vi "Microscope_control-illumination_camera_Galvo_EOM.vi"() -> ()   [LabVIEW 2012]
uses:
  <vilib>/Utility/error.llb/DialogType.ctl
  <vilib>/DAQmx/read.llb/DAQmx Read (Analog DBL 1Chan 1Samp).vi
  <vilib>/DAQmx/write.llb/DAQmx Write (Digital 1D Bool NChan 1Samp 1Line).vi
  <vilib>/DAQmx/write.llb/DAQmx Write (Analog 1D DBL NChan 1Samp).vi
  <vilib>/DAQmx/read.llb/DAQmx Read (Analog 2D DBL NChan NSamp).vi
  <vilib>/DAQmx/write.llb/DAQmx Write (Analog 1D Wfm NChan NSamp).vi
  <vilib>/DAQmx/write.llb/DAQmx Write (Analog DBL 1Chan 1Samp).vi
  <vilib>/DAQmx/create/channels.llb/DAQmx Create Channel (AI-Voltage-Basic).vi
  <vilib>/DAQmx/miscellaneous.llb/DAQmx Fill In Error Info.vi
  <vilib>/addons/control/pid/pid.llb/PID Advanced (DBL).vi
  <vilib>/DAQmx/create/channels.llb/DAQmx Create Channel (DO-Digital Output).vi
  <vilib>/DAQmx/create/channels.llb/DAQmx Create Channel (AO-Voltage-Basic).vi
  <vilib>/Analysis/baseanly.llb/Mean (DBL).vi
  <vilib>/DAQmx/configure/timing.llb/DAQmx Timing (Use Waveform).vi
  <vilib>/Analysis/NI_AALBase.lvlib
  <instrlib>/Olympus IX BX Series/Olympus IX BX Series.lvlib
  <vilib>/addons/control/pid/NI_PID_pid.lvlib
panel:
  in  "Laser Trig 1":bool
  in  "# repeats":i16=6
  in  "Splice?":bool
  in  "Digital  Time Step":dbl=0.0005 format="%.4f"
  in  "Synced Trigger?":bool
  out "Digital Waveform":digitalwaveform[](graph)=[{"t0"=timestamp(0 s since 1904-01-01), "dt"=0.0, "Y"={"transitions"=[0, 2, 30, 32, 60, 62, 90, 92, 120, 122, 150, 152, 180, 182, 210, 212, 240, 242, 270, 272, 300, 302, 330, 332, 360, 362, 390, 392, 420, 422, 450, 452, 480, 482, 510, 512, 540, 542, 570, 572, 600, 601], "data"=[[1], [0], [1], [0], [1], [0], [1], [0], [1], [0], [1], [0], [1], [0], [1], [0], [1], [0], [1], [0], [1], [0], [1], [0], [1], [0], [1], [0], [1], [0], [1], [0], [1], [0], [1], [0], [1], [0], [1], [0], [1], [0]]}, "error"={"status"=FALSE, "code"=37421928, "source"=""}}, {"t0"=timestamp(0 s since 1904-01-01), "dt"=0.0, "Y"={"transitions"=[0, 11, 21, 41, 51, 71, 81, 101, 111, 131, 141, 161, 171, 191, 201, 221, 231, 251, 261, 281, 291, 311, 321, 341, 351, 371, 381, 401, 411, 431, 441, 461, 471, 491, 501, 521, 531, 551, 561, 581, 591, 601], "data"=[[0], [1], [0], [1], [0], [1], [0], [1], [0], [1], [0], [1], [0], [1], [0], [1], [0], [1], [0], [1], [0], [1], [0], [1], [0], [1], [0], [1], [0], [1], [0], [1], [0], [1], [0], [1], [0], [1], [0], [1], [0], [0]]}, "error"={"status"=FALSE, "code"=37421928, "source"=""}}]
  out "number of samples":i32=602
  in  "CO.Pulse.Term":tag="/Dev2/PFI0"
  in  "Cycle time":dbl=30.0 format="%.4f"
  out "Clock Rate":dbl=66666.66666666667
  in  "Digital lines":tag="Dev2/port0/line8:9"
  in  "Digital Data":digitalwaveform[](array[waveform])=[{"t0"=timestamp(0 s since 1904-01-01), "dt"=0.0, "Y"={"transitions"=[0, 2, 30, 32, 60, 62, 90, 92, 120, 122, 150, 152, 180, 182, 210, 212, 240, 242, 270, 272, 300, 302, 330, 332, 360, 362, 390, 392, 420, 422, 450, 452, 480, 482, 510, 512, 540, 542, 570, 572, 600, 601], "data"=[[1], [0], [1], [0], [1], [0], [1], [0], [1], [0], [1], [0], [1], [0], [1], [0], [1], [0], [1], [0], [1], [0], [1], [0], [1], [0], [1], [0], [1], [0], [1], [0], [1], [0], [1], [0], [1], [0], [1], [0], [1], [0]]}, "error"={"status"=FALSE, "code"=37421928, "source"=""}}, {"t0"=timestamp(0 s since 1904-01-01), "dt"=0.0, "Y"={"transitions"=[0, 11, 21, 41, 51, 71, 81, 101, 111, 131, 141, 161, 171, 191, 201, 221, 231, 251, 261, 281, 291, 311, 321, 341, 351, 371, 381, 401, 411, 431, 441, 461, 471, 491, 501, 521, 531, 551, 561, 581, 591, 601], "data"=[[0], [1], [0], [1], [0], [1], [0], [1], [0], [1], [0], [1], [0], [1], [0], [1], [0], [1], [0], [1], [0], [1], [0], [1], [0], [1], [0], [1], [0], [1], [0], [1], [0], [1], [0], [1], [0], [1], [0], [1], [0], [0]]}, "error"={"status"=FALSE, "code"=37421928, "source"=""}}]
  in  "counter ch. #":tag="Dev2/ctr0"
  out "Array":dbl[](array[numeric])=[5.218535567851096e-05]
  in  "Quiver full amp":dbl=10.0 min=0.0 max=360.0 format="%0.1p"
  in  "W-E Phase":dbl format="%.2f"
  in  "Quiver Direction":i32(ring) items=["North", "East", "South", "West"]
  in  "quiver offset":dbl format="%0.2p"
  in  "quiver offset":dbl format="%0.2p"
  in  "EOM spin? (Quiver)":bool
  in  "Phase":dbl format="%.2f"
  in  "Phase":dbl step=0.1 format="%.2f"
  in  "Offset":dbl min=-1.0 max=1.0 step=0.001 format="%.3f"
  in  "Offset":dbl min=-1.0 max=1.0 format="%.3f"
  out "Quivering":bool
  in  "180° Shift":bool
  in  "180° Shift":bool
  in  "Quiver":bool
  in  "180° Shift":bool
  in  "180° Shift (s)":bool
  in  "Center exclude":dbl=0.1
  in  "E/W EOM":dbl=0.07
  in  "N/S EOM":dbl=0.07
  in  "EOM spin?":bool=TRUE
  in  "EOM Voltage (Ch. 3)":dbl(slide) step=0.0001 scale=-0.7..0.7 scale format="%#_4g"
  out "Direction":u16(ring) items=["", "North", "East", "South", "West", "Spin", "Sync"]
  in  "Center":bool
  in  "South":bool
  in  "East":bool
  in  "West":bool
  in  "North":bool
  in  "output range":cluster{"out high":dbl, "out low":dbl}={"out high"=1.0, "out low"=-1.0} {"out low" format="%.2f"; "out high" format="%.2f"}
  in  "Lock-in Amp In":tag="Dev2/ai16" caption="Lock In Detect In"
  in  "Focus Position?":bool
  out "position (um)":T1(graph)={"data"=-0.13365967335514356, "position (um)"=7583.27, "element"=0.0}
  in  "Use current position?":bool
  in  "setpoint range":cluster{"SP high":dbl, "SP low":dbl}={"SP high"=5.0, "SP low"=-5.0} {"SP high" format="%.2f"; "SP low" format="%.2f"}
  out "Notification":u16(ring) items=["", "Spin must be activated for focus lock", "Spin must be activated for focus detection", "Disable EOM spin"]
  in  "Lock Z":bool
  in  "Focus limit width":dbl=1000.0
  in  "Focus Limit Center":dbl=7500.0 format="%.1f"
  in  "IX2-UCB port":refnum<visa-resource-name>="COM1"
  in  "Sampling Time":dbl=100.0 format="%.2f"
  in  "PID gains":T2={"proportional gain (Kc)"=0.8, "integral time (Ti, min)"=0.0, "derivative time (Td, min)"=0.0} {"derivative time (Td, min)" format="%#.6g"; "integral time (Ti, min)" format="%#.6g"; "proportional gain (Kc)" format="%#.6g"}
  in  "Z lock setpoint (Volt)":dbl(slide) min=-5.0 max=5.0 step=0.01 scale=-5.0..5.0 scale format="%#_4g"
  in  "Write Y/X ration \nduring center find?":bool=TRUE
  out "W-E Width":dbl=0.63 format="%#_5g"
  out "N-S Width":dbl=0.63 format="%#_5g"
  out "Spinning":bool
  in  "Stop spin":bool caption="stop"
  out "output cluster":cluster{dbl, "# sample":i32}={66666.66666666667, "# sample"=2000}
  in  "# sample":i32=2000
  in  "Y/X ration \nW-E = C*(N-S)":dbl=1.0 format="%.3f"
  in  "Amplitude":dbl min=0.0 max=1.0 step=0.001 format="%.3f"
  in  "Amplitude":dbl=-0.54 step=0.001 format="%.3f"
  in  "Offset":dbl min=-1.0 max=1.0 format="%.3f"
  in  "Offset":dbl=-0.135 min=-1.0 max=1.0 step=0.001 format="%.3f"
  out "Output Waveform":waveform(dbl)[](graph)=[{"t0"=timestamp(0 s since 1904-01-01), "dt"=1.4999999999999999e-05, "Y"=array[2000 elements]}, {"t0"=timestamp(0 s since 1904-01-01), "dt"=1.4999999999999999e-05, "Y"=array[2000 elements]}, {"t0"=timestamp(0 s since 1904-01-01), "dt"=1.4999999999999999e-05, "Y"=array[2000 elements]}, {"t0"=timestamp(0 s since 1904-01-01), "dt"=1.4999999999999999e-05, "Y"=array[2000 elements]}]
  in  "Spin Amp (N-S)":dbl=0.68 format="%.3f"
  in  "Phase":dbl step=0.1 format="%.2f"
  in  "Phase":dbl=-70.0 format="%.2f"
  in  "W-E Phase Delay":dbl=90.0 format="%.2g"
  in  "Frequency":dbl=200.0 min=0.0 max=300.0 format="%0.2p"
  in  "Spin":bool
  out "Text Ring":u16(ring)=1 items=["East-West", "North-South"]
  in  "Centering Iterations":i32=4
  in  "2D Center Find":bool
  in  "Y":dbl(slide) scale=1.0..-1.0 scale format="%#.4g"
  in  "X":dbl(slide) scale=-1.0..1.0 scale format="%#.3g"
  out "Manual Control":dbl(knob)=-0.003845687659202201 scale=-0.01..0.2
  in  "Differential Initial Conditions":dbl[](array[numeric])=[-0.005, -0.005] format="%#_6f"
  in  "Scan Galvo Selection":bool
  out "Amplitude":dbl=0.63 format="%#_4g"
  out "Offset":dbl=0.03399999999999992 format="%#_3g"
  out "Right":dbl=0.6639999999999999 format="%#_4g"
  out "left":dbl=-0.5960000000000001 format="%#_4g"
  in  "Differential Method":u16(ring)=1 items=["2nd Order Central", "4th Order Central", "Forward", "Backward"]
  out "X Y Sensor Graph":cluster{"Array":dbl[], "Array":dbl[]}[](graph)
  in  "samples per step":i32=10
  out "Sum Graph":cluster{"Array":dbl[], "dX/dt":dbl[]}[](graph)
  in  "Analog Input Channels":tag="Dev2/ai0:2" caption="Quad Detector In"
  in  "ms to wait":u32
  in  "Steps":i16=1601 caption="scan steps"
  in  "End voltage (scanned galvo)":dbl=0.8 caption="End Scan" format="%0.2f"
  in  "Start voltage (scanned galvo)":dbl=-0.8 caption="Start Scan" format="%0.2f"
  in  "Galvo Hard Max Voltage":dbl=1.0 caption="Max Value" format="%0.2f"
  in  "Galvo Hard Min Voltage":dbl=-1.0 caption="Min Value" format="%0.2f"
  in  "Analog Out Channels":tag="Dev2/ao0:3" caption="Galvo/EOM Out"
  in  "Scan Galvo":bool
  in  "stop":bool
  # "N-S"
  # "E-W"
  # "Channel 3"
  # "Channel 4"
  # "Channel 3"
  # "Channel 4"
  # "Hz"
  # "deg"
  # "V"
  # "deg"
  # "N"
  # "s"
  # "s"
  # "N/S (p), \nE/W (s)"
  # "N/S (s), \nE/W (p)"
  # "W"
  # "E"
  # "S"
  # "V"
  # "V"
  # "N/S (p), \nE/W (s)"
  # "DAQ Parameters"
  # "ms"
  # "nm"
  # "nm"
  # "Center Scan Parameters"
  # "V"
  # "V"
  # "V"
  # "ms"
  # "V"
  # "Notes: Analog Output Ch. 1 and 2 designed to control two axis of galvonometers, Ch.3 and 4 are for EOM. \nCh.1 and 2 consists of sine wave, typically with relative phase shift of ~90 deg, to generate a circular scan\nCh. 3 and 4 are sawtooth scans at twice frequency of Ch. 1 and 2.  \n2D centerfind detects X and Y axis TIR conditions (from back reflection detector), in order to find beam center position for circle scanning\nParameters on upper right panels are for sending TTL pulses/triggers to lasers/cameras/flow valves.  Ch. 1-4 analog outputs (for galvos and EOM) can be synced with this TTL triggers\nParameters on lower right are for controlling microscope focus feedback using back reflection detector (Olympus IX2 series)."
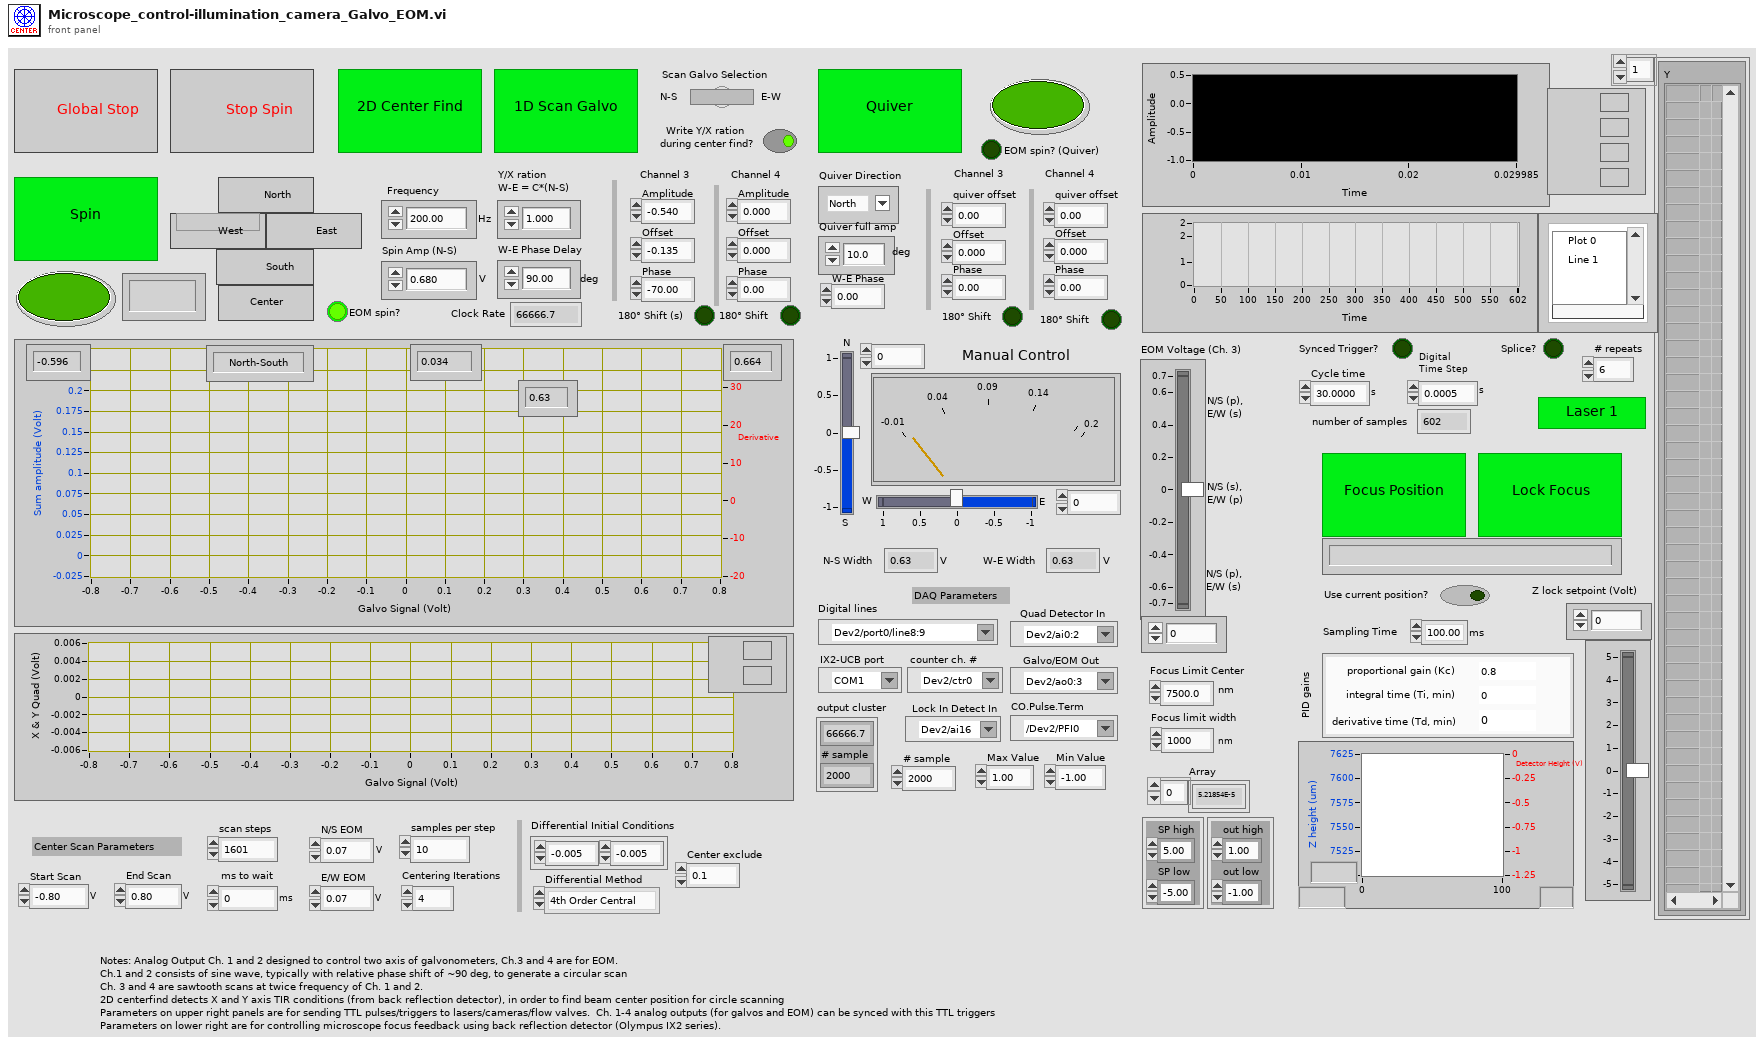
[diagram p1: front panel]
types:
  T1 = cluster{"data":dbl, "position (um)":dbl, "element":dbl}
  T2 = cluster{"proportional gain (Kc)":dbl, "integral time (Ti, min)":dbl, "derivative time (Td, min)":dbl}
  T3 = typedef "DialogType.ctl" = u16
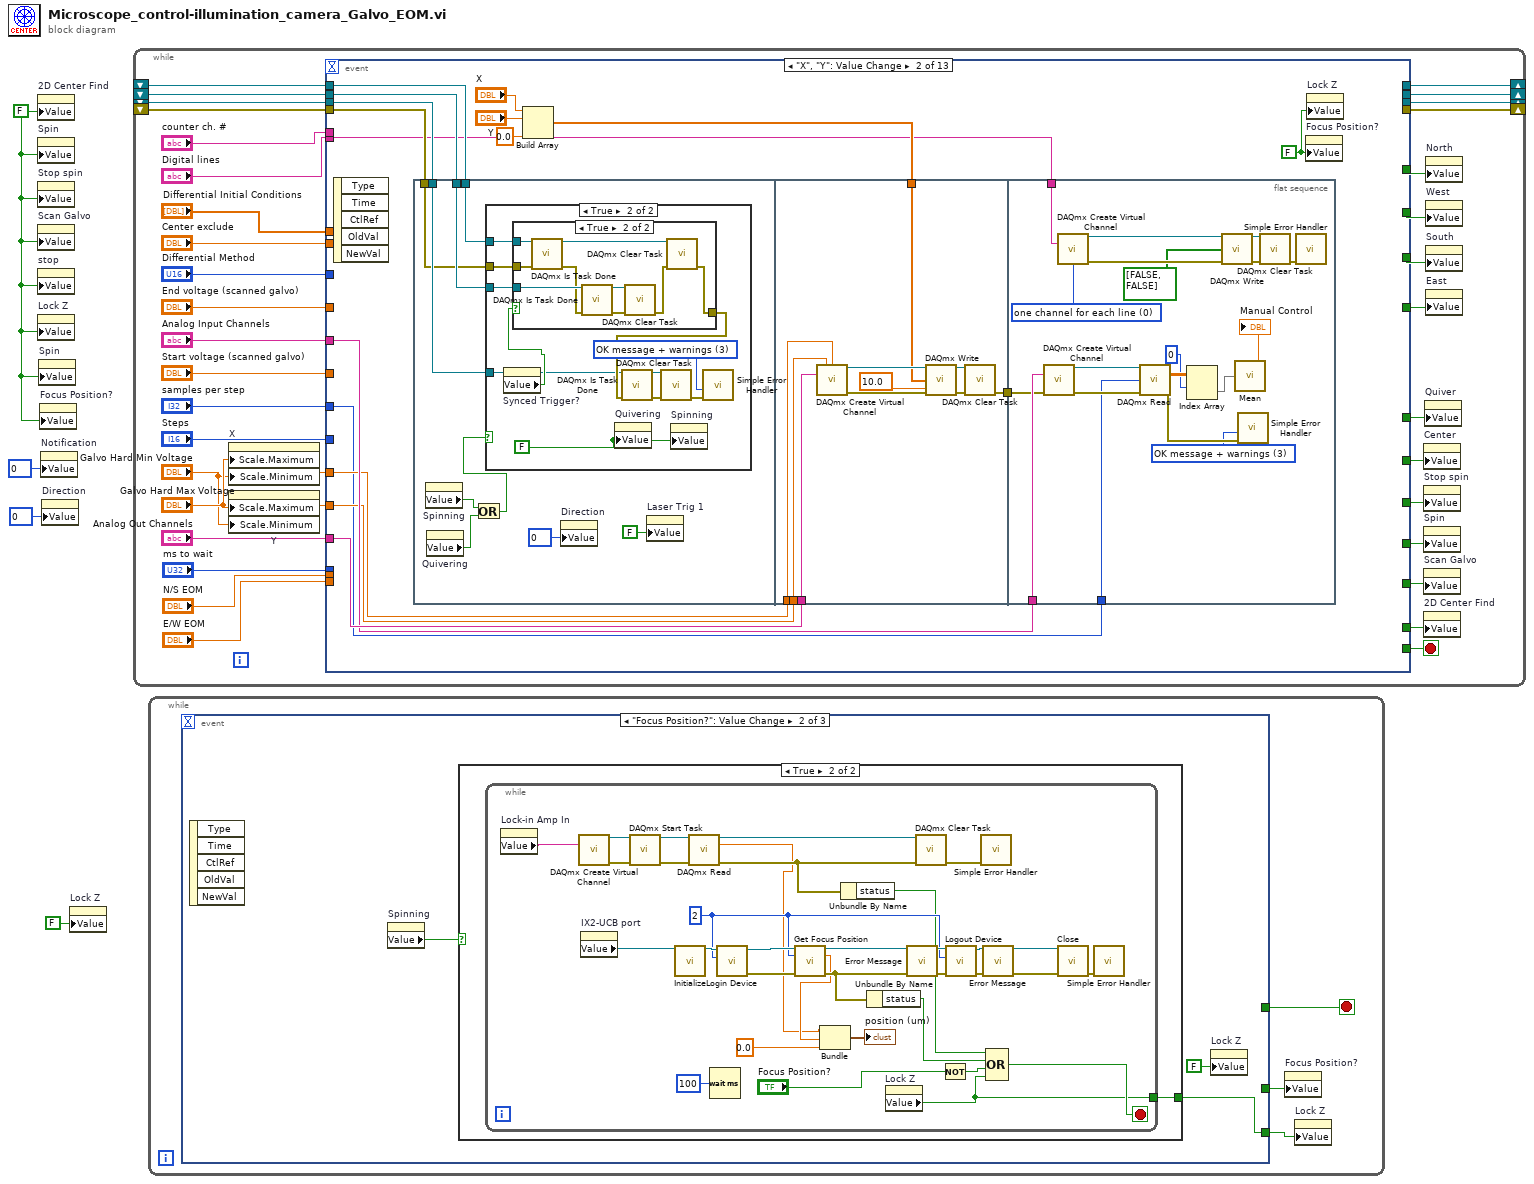
[diagram p0: block diagram]
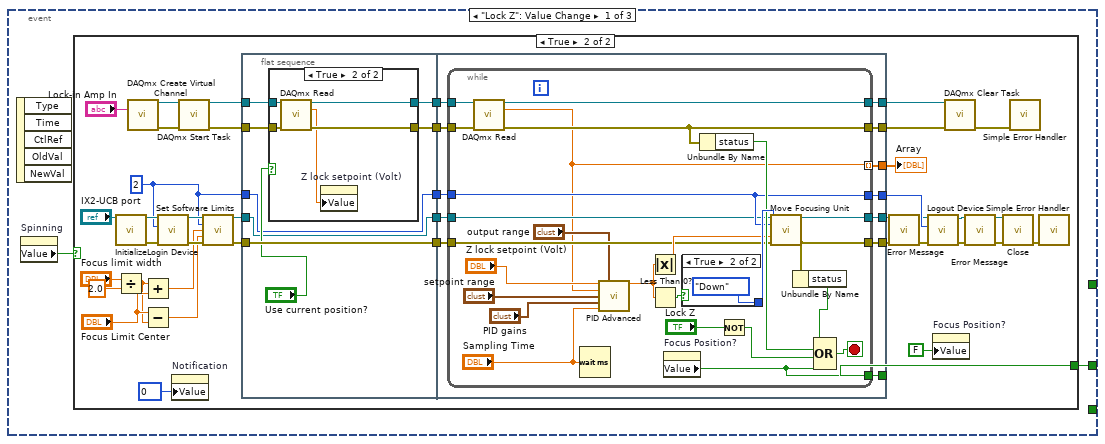
[diagram p2: hidden frame]
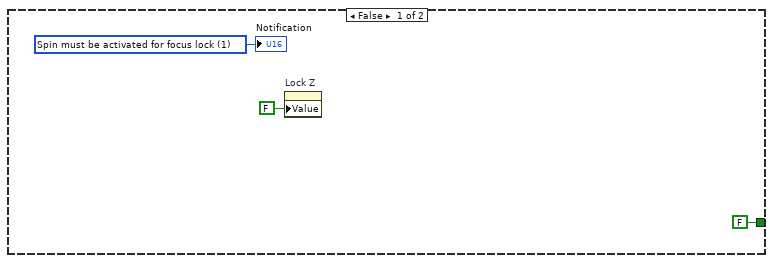
[diagram p3: hidden frame]
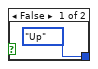
[diagram p5: hidden frame]
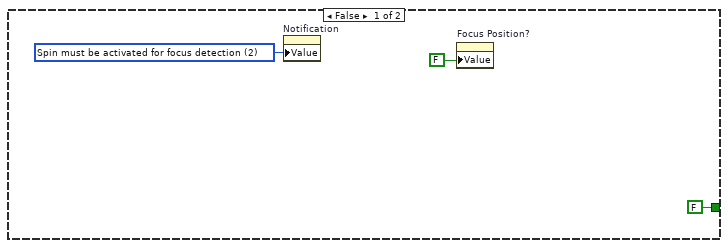
[diagram p6: hidden frame]
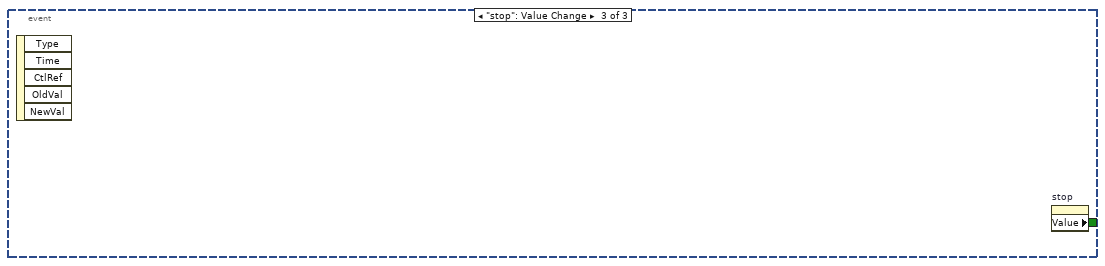
[diagram p7: hidden frame]
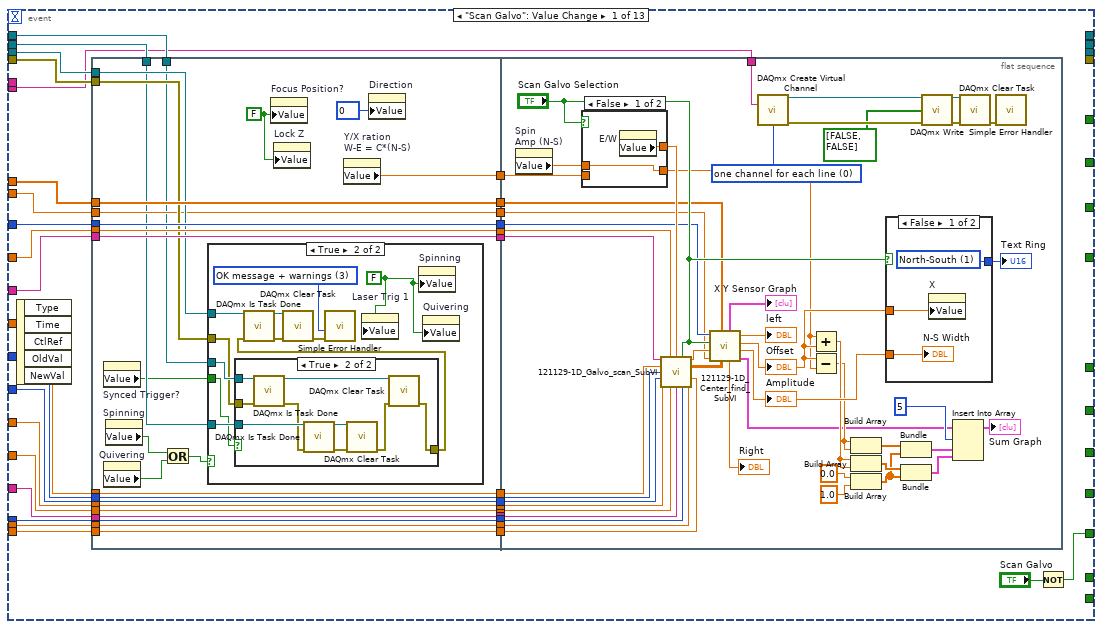
[diagram p8: hidden frame]
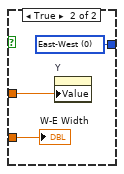
[diagram p11: hidden frame]
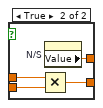
[diagram p12: hidden frame]
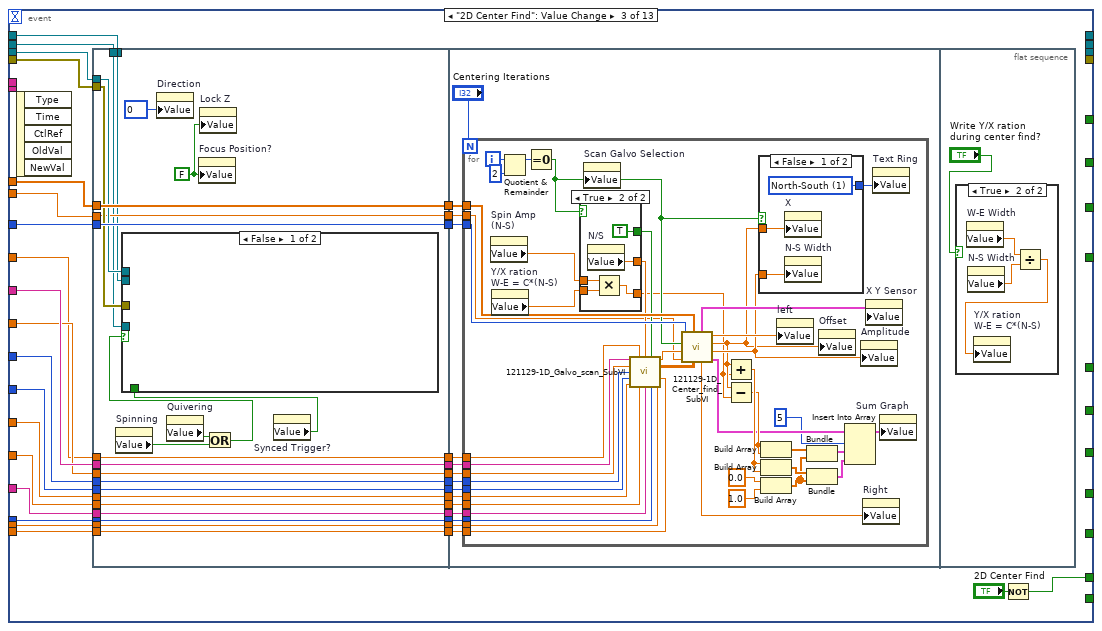
[diagram p15: hidden frame]
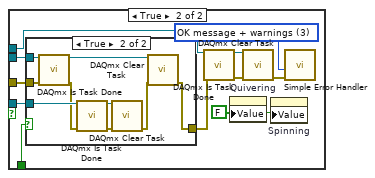
[diagram p16: hidden frame]
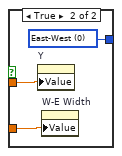
[diagram p18: hidden frame]
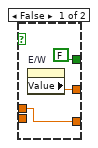
[diagram p19: hidden frame]
diagram:
  w2 = u16 0 items=["", "North", "East", "South", "West"] ("Direction")
  w4 = u16 0 items=["", "Active spin for focus lock"] ("Text Ring 2")
  w1 = FALSE ("2D Center Find")
  n1 = property on="2D Center Find" class="Bool (strict)"("Value"=w1) -> ()  [unwired: 2 in, 2 out]
  n2 = property on="Spin" class="Bool (strict)"("Value"=w1) -> ()  [unwired: 2 in, 2 out]
  n3 = property on="Stop spin" class="Bool (strict)"("Value"=w1) -> ()  [unwired: 2 in, 2 out]
  n4 = property on="Scan Galvo" class="Bool (strict)"("Value"=w1) -> ()  [unwired: 2 in, 2 out]
  n5 = property on="stop" class="Bool (strict)"("Value"=w1) -> ()  [unwired: 2 in, 2 out]
  n6 = property on="Lock Z" class="Bool (strict)"("Value"=w1) -> ()  [unwired: 2 in, 2 out]
  n7 = property on="Spin" class="Bool (strict)"("Value"=w1) -> ()  [unwired: 2 in, 2 out]
  n8 = property on="Focus Position?" class="Bool (strict)"("Value"=w1) -> ()  [unwired: 2 in, 2 out]
  n9 = property on="Notification" class="Ring (strict)"("Value"=w4) -> ()  [unwired: 2 in, 2 out]
  n10 = property on="Direction" class="Ring (strict)"("Value"=w2) -> ()  [unwired: 2 in, 2 out]
  n11 = property on="Lock Z" class="Bool (strict)"("Value"=FALSE ("Lock Z")) -> ()  [unwired: 2 in, 2 out]
  n12 = while {
    shift-right: [w25] -> _
    shift-left: _ -> [w23]
    shift-right: [w24] -> _
    shift-left: _ -> [w22]
    shift-right: [w10] -> _
    shift-left: _ -> [w8]
    shift-right: [w9] -> _
    shift-left: _ -> [w7]
    stop <- w39 stop-if-true
    n13 = property on="X" class="Slide (strict)"("Scale.Maximum"="Galvo Hard Max Voltage", "Scale.Minimum"="Galvo Hard Min Voltage") -> ()  [unwired: 2 in, 2 out]
    n14 = property on="Y" class="Slide (strict)"("Scale.Maximum"="Galvo Hard Max Voltage", "Scale.Minimum"="Galvo Hard Min Voltage") -> ()  [unwired: 2 in, 2 out]
    n15 = event shown="[1] \"X\", \"Y\": Value Change" {
      selector: _ -> [_ _ _ _ _ _ _ _ _ _ _ _ _]
      dyn-events: _ -> [_ _ _ _ _ _ _ _ _ _ _ _ _]
      timeout: _ -> [_ _ _ _ _ _ _ _ _ _ _ _ _]
      tunnel: [_ _ _ _ _ _ _ _ _ _ _ _ "stop"] -> w39
      tunnel: [w74 _ _ _ _ _ _ _ _ _ _ _ _] -> w38
      tunnel: "Galvo Hard Max Voltage" -> [w73 w191 w282 _ _ w681 w746 w812 w877 _ _ w997 w1060]
      tunnel: "Galvo Hard Min Voltage" -> [w72 w192 w283 _ _ w680 w747 w813 w878 _ _ w996 w1059]
      tunnel: "Analog Out Channels" -> [w71 w195 w281 w420 w549 w682 w745 w811 w876 w941 _ w995 w1061]
      tunnel: "Analog Input Channels" -> [w70 w194 w287 _ _ _ _ _ _ _ _ _ _]
      tunnel: "samples per step" -> [w69 w190 w285 _ _ _ _ _ _ _ _ _ _]
      tunnel: [_ _ w288 _ _ _ _ _ _ _ _ _ _] -> w32
      tunnel: "Steps" -> [w68 _ w284 _ _ _ _ _ _ _ _ _ _]
      tunnel: "End voltage (scanned galvo)" -> [w67 _ w279 _ _ _ _ _ _ _ _ _ _]
      tunnel: "Start voltage (scanned galvo)" -> [w66 _ w286 _ _ _ _ _ _ _ _ _ _]
      tunnel: "Differential Method" -> [w65 _ w278 _ _ _ _ _ _ _ _ _ _]
      tunnel: "Differential Initial Conditions" -> [w64 _ w277 _ _ _ _ _ _ _ _ _ _]
      tunnel: "ms to wait" -> [w63 _ w280 _ _ _ _ _ _ _ _ _ _]
      tunnel: [_ _ _ w425 w552 _ _ _ _ w943 w976 _ _] -> w25
      tunnel: [_ _ _ w424 w551 _ _ _ _ w942 w968 _ _] -> w24
      tunnel: w23 -> [w51 w186 w265 w412 w553 w683 w748 w815 w880 w943 w976 w998 w1062]
      tunnel: w22 -> [w50 w187 w264 w416 w554 w675 w740 w814 w879 w942 w969 w988 w1055]
      tunnel: [_ _ _ _ _ _ _ _ _ _ _ FALSE _] -> w21
      tunnel: [_ _ _ w422 _ _ _ _ _ _ _ _ _] -> w20
      tunnel: [_ _ _ _ _ _ _ _ _ _ _ FALSE _] -> w19
      tunnel: [_ _ _ _ _ _ _ _ w875 _ _ _ _] -> w18
      tunnel: [_ _ _ _ _ _ _ w809 _ _ _ _ _] -> w17
      tunnel: [_ _ _ _ _ _ w744 _ _ _ _ _ _] -> w16
      tunnel: [_ _ _ _ _ w678 _ _ _ _ _ _ _] -> w15
      tunnel: "N/S EOM" -> [w48 _ w262 _ _ _ _ _ _ _ _ _ _]
      tunnel: "E/W EOM" -> [w46 _ w261 _ _ _ _ _ _ _ _ _ _]
      tunnel: "Center exclude" -> [w43 _ w258 _ _ _ _ _ _ _ _ _ _]
      tunnel: [_ _ _ _ w550 _ _ _ _ _ _ _ _] -> w11
      tunnel: [_ _ _ w418 _ _ _ _ _ w939 _ _ _] -> w10
      tunnel: [_ _ _ w417 _ _ _ _ _ w938 _ _ _] -> w9
      tunnel: w8 -> [w42 w183 w257 w415 w548 w677 w742 w807 w872 w939 w972 w990 w1057]
      tunnel: w7 -> [w41 w182 w256 w414 w547 w676 w741 w806 w871 w938 w971 w989 w1056]
      tunnel: "Digital lines" -> [w40 w181 _ w413 w546 w674 w739 w808 w873 _ w967 w987 w1054]
      tunnel: "counter ch. #" -> [_ _ _ w411 _ _ _ _ _ _ _ _ _]
      event "Scan Galvo": Value Change {
        n16 = event-data() -> ()  [unwired: 1 in, 5 out]
        n17 = flat-sequence {
          tunnel: w63 -> [w90]
          tunnel: w64 -> [w91]
          tunnel: w65 -> [w92]
          tunnel: w66 -> [w93]
          tunnel: w67 -> [w94]
          tunnel: w68 -> [w95]
          tunnel: w69 -> [w96]
          tunnel: w70 -> [w97]
          tunnel: w71 -> [w98]
          tunnel: w72 -> [w99]
          tunnel: w73 -> [w100]
          tunnel: [w100] -> w62
          tunnel: [w99] -> w61
          tunnel: [w98] -> w60
          tunnel: [w97] -> w59
          tunnel: [w96] -> w58
          tunnel: [w95] -> w57
          tunnel: [w94] -> w56
          tunnel: [w93] -> w55
          tunnel: [w92] -> w54
          tunnel: [w91] -> w53
          tunnel: [w90] -> w52
          tunnel: w51 -> [w89]
          tunnel: w50 -> [w88]
          tunnel: [w87] -> w49
          tunnel: w48 -> [w85]
          tunnel: [w85] -> w47
          tunnel: w46 -> [w84]
          tunnel: [w84] -> w45
          tunnel: w43 -> [w83]
          tunnel: [w83] -> w44
          tunnel: w42 -> [w79]
          tunnel: w41 -> [w78]
          tunnel: w62 -> [w163]
          tunnel: w61 -> [w162]
          tunnel: w60 -> [w161]
          tunnel: w59 -> [w160]
          tunnel: w58 -> [w159]
          tunnel: w57 -> [w156]
          tunnel: w56 -> [w155]
          tunnel: w55 -> [w154]
          tunnel: w54 -> [w153]
          tunnel: w53 -> [w152]
          tunnel: w52 -> [w151]
          tunnel: w49 -> [w133]
          tunnel: w47 -> [w131]
          tunnel: w45 -> [w132]
          tunnel: w44 -> [w130]
          tunnel: w40 -> [w122]
          frame #0 {
            w86 = u16 0 items=["", "North", "East", "South", "West"] ("Direction")
            w76 = FALSE ("Focus Position?")
            n18 = property on="Synced Trigger?" class="Bool (strict)"() -> ("Value"=w77:bool)  [unwired: 2 in, 2 out]
            n19 = property on="Quivering" class="Bool (strict)"() -> ("Value"=w81:bool)  [unwired: 2 in, 2 out]
            n20 = property on="Spinning" class="Bool (strict)"() -> ("Value"=w82:bool)  [unwired: 2 in, 2 out]
            n21 = Or(x=w82, y=w81) -> (x .or. y?=w80:bool)
            n22 = case shown="True" w80 {
              tunnel: w89 -> [_ w107]
              tunnel: w88 -> [_ w104]
              tunnel: w79 -> [_ w106]
              tunnel: w78 -> [_ w105]
              tunnel: w77 -> [_ w102]
              frame False {
              }
              frame True {
                w101 = FALSE ("Spinning")
                w111 = T3 3 items=["no dialog", "OK message", "continue or stop message", "OK message + warnings", "continue/stop + warnings"] ("type of dialog (OK msg:1)")
                n23 = case shown="True" w102 {
                  tunnel: w106 -> [_ w121]
                  tunnel: w105 -> [_ w120]
                  tunnel: w104 -> [w112 w119]
                  tunnel: [w112 w113] -> w103
                  frame False {
                  }
                  frame True {
                    n24 = call <vilib>:"DAQmx Is Task Done.vi"("task/channels in"=w121, "error in"=w119) -> ("task out"=w114:refnum<k21>, "error out"=w118:errorcluster)  [unwired: 11 in, 1 out]
                    n25 = call <vilib>:"DAQmx Is Task Done.vi"("task/channels in"=w120, "error in"=w118) -> ("task out"=w116:refnum<k21>, "error out"=w117:errorcluster)  [unwired: 11 in, 1 out]
                    n26 = call <vilib>:"DAQmx Clear Task.vi"("task in"=w116, "error in"=w117) -> ("error out"=w115:errorcluster)  [unwired: 13 in]
                    n27 = call <vilib>:"DAQmx Clear Task.vi"("task in"=w114, "error in"=w115) -> ("error out"=w113:errorcluster)  [unwired: 13 in]
                  }
                }
                n28 = call <vilib>:"DAQmx Is Task Done.vi"("task/channels in"=w107, "error in"=w103) -> ("task out"=w108:refnum<k21>, "error out"=w109:errorcluster)  [unwired: 11 in, 1 out]
                n29 = call <vilib>:"DAQmx Clear Task.vi"("task in"=w108, "error in"=w109) -> ("error out"=w110:errorcluster)  [unwired: 13 in]
                n30 = call <vilib>:"Simple Error Handler.vi"("type of dialog (OK msg:1)"=w111, "error in (no error)"=w110) -> ()  [unwired: 3 in, 5 out]
                n31 = property on="Laser Trig 1" class="Bool (strict)"("Value"=w101) -> ()  [unwired: 2 in, 2 out]
                n32 = property on="Spinning" class="Bool (strict)"("Value"=w101) -> ()  [unwired: 2 in, 2 out]
                n33 = property on="Quivering" class="Bool (strict)"("Value"=w101) -> ()  [unwired: 2 in, 2 out]
              }
            }
            n34 = property on="Focus Position?" class="Bool (strict)"("Value"=w76) -> ()  [unwired: 2 in, 2 out]
            n35 = property on="Lock Z" class="Bool (strict)"("Value"=w76) -> ()  [unwired: 2 in, 2 out]
            n36 = property on="Y/X ration \nW-E = C*(N-S)" class="DigNum (strict)"() -> ("Value"=w87:dbl)  [unwired: 2 in, 2 out]
            n37 = property on="Direction" class="Ring (strict)"("Value"=w86) -> ()  [unwired: 2 in, 2 out]
          }
          frame #1 {
            w124 = 0 items=["one channel for each line", "one channel for all lines"] ("line grouping")
            n38 = property on="Spin \nAmp (N-S)" class="DigNum (strict)"() -> ("Value"=w135:dbl)  [unwired: 2 in, 2 out]
            n39 = case shown="False" "Scan Galvo Selection" {
              tunnel: [w176 w180] -> w158
              tunnel: w135 -> [w175 w178]
              tunnel: [w175 w179] -> w134
              tunnel: w133 -> [_ w177]
              frame False {
                n40 = property on="E/W" class="Slide (strict)"() -> ("Value"=w176:dbl)  [unwired: 2 in, 2 out]
              }
              frame True {
                n41 = Multiply(x=w178, y=w177) -> (x*y=w179:dbl)
                n42 = property on="N/S" class="Slide (strict)"() -> ("Value"=w180:dbl)  [unwired: 2 in, 2 out]
              }
            }
            n43 = call "121129-1D_Galvo_scan_SubVI.vi"("Analog Input Channels"=w160, "End voltage (scanned galvo)"=w155, "Voltage (fixed galvo)"=w158, "Scan Galvo Selection"="Scan Galvo Selection", "Start voltage (scanned galvo)"=w154, "number of samples per channel"=w159, "Steps"=w156, "E/W EOM"=w132, "Galvo Hard Min Voltage"=w162, "Galvo Hard Max Voltage"=w163, "Analog Out Channels"=w161, "milliseconds to wait"=w151, "N/S EOM"=w131) -> ("Delta V spacing"=w167:dbl, "Array"=w164:dbl[][])  [unwired: 1 in]
            n44 = call "121129-1D_Center_find_SubVI.vi"("Array in"=w164, "Differential Initial Conditions"=w152, "Center exclude"=w130, "Delta V spacing"=w167, "Scan Galvo Selection"="Scan Galvo Selection", "Differential Method"=w153) -> ("Sum Graph"=w137:cluster{"Array":dbl[], "dX/dt":dbl[]}[], "Amplitude"=w149:dbl, "Offset"=w139:dbl, "left"=→"left":dbl, "Right"=→"Right":dbl, "X Y Sensor Graph"=→"X Y Sensor Graph":cluster{"Array":dbl[], "Array":dbl[]}[])
            "Offset" <- w139
            "Amplitude" <- w149
            n45 = call-poly <vilib>:"DAQmx Create Virtual Channel.vi"("lines"=w122, "line grouping"=w124) -> ("task out"=w129:refnum<k21>, "error out"=w128:errorcluster)  [unwired: 12 in]
            n46 = Add(x=w134, y=w139) -> (x+y=w144:dbl)
            n47 = Subtract(x=w139, y=w134) -> (x-y=w138:dbl)
            n48 = Build Array(w138, w138) -> (w140:dbl[])
            n49 = Build Array(w144, w144) -> (w145:dbl[])
            n50 = Build Array(0.0 ("element"), 1.0 ("element")) -> (w141:dbl[])
            n51 = case shown="False" "Scan Galvo Selection" {
              tunnel: w139 -> [w171 w174]
              tunnel: [w170 w173] -> w150
              tunnel: w149 -> [w169 w172]
              frame False {
                w170 = u16 1 items=["East-West", "North-South"] ("Text Ring")
                n52 = property on="X" class="Slide (strict)"("Value"=w171) -> ()  [unwired: 2 in, 2 out]
                "N-S Width" <- w169
              }
              frame True {
                w173 = u16 0 items=["East-West", "North-South"] ("Text Ring")
                n53 = property on="Y" class="Slide (strict)"("Value"=w174) -> ()  [unwired: 2 in, 2 out]
                "W-E Width" <- w172
              }
            }
            "Text Ring" <- w150
            n54 = Bundle(w140, w141) -> (w142:cluster{dbl[], dbl[]})  [unwired: 1 in]
            n55 = Bundle(w145, w141) -> (w143:cluster{dbl[], dbl[]})  [unwired: 1 in]
            n56 = call-poly <vilib>:"DAQmx Write.vi"("task/channels in"=w129, "data"=bool[] [FALSE, FALSE], "error in"=w128) -> ("task out"=w126:refnum<k21>, "error out"=w127:errorcluster)  [unwired: 10 in, 1 out]
            n57 = Insert Into Array(array=w137, index=5, new element #1=w142, new element #2=w143) -> (→"Sum Graph":cluster{"Array":dbl[], "dX/dt":dbl[]}[])
            n58 = call <vilib>:"DAQmx Clear Task.vi"("task in"=w126, "error in"=w127) -> ("error out"=w125:errorcluster)  [unwired: 13 in]
            n59 = call <vilib>:"Simple Error Handler.vi"("error in (no error)"=w125) -> ()  [unwired: 4 in, 5 out]
          }
        }
        n60 = Not(x="Scan Galvo") -> (.not. x?=w74:bool)
      }
      event "X", "Y": Value Change {
        w184 = FALSE ("Focus Position?")
        w185 = 0.0 ("element")
        n61 = event-data() -> ()  [unwired: 1 in, 5 out]
        n62 = flat-sequence {
          tunnel: w187 -> [w198]
          tunnel: w186 -> [w205]
          tunnel: w183 -> [w200]
          tunnel: w182 -> [w199]
          tunnel: w195 -> [w231]
          tunnel: w196 -> [w230]
          tunnel: [w229] -> w193
          tunnel: w192 -> [w228]
          tunnel: w191 -> [w227]
          tunnel: w194 -> [w251]
          tunnel: w193 -> [w249]
          tunnel: w190 -> [w246]
          tunnel: w181 -> [w237]
          frame #0 {
            w204 = u16 0 items=["", "North", "East", "South", "West"] ("Direction")
            n63 = property on="Spinning" class="Bool (strict)"() -> ("Value"=w202:bool)  [unwired: 2 in, 2 out]
            n64 = property on="Quivering" class="Bool (strict)"() -> ("Value"=w203:bool)  [unwired: 2 in, 2 out]
            n65 = Or(x=w202, y=w203) -> (x .or. y?=w201:bool)
            n66 = case shown="True" w201 {
              tunnel: w205 -> [_ w207]
              tunnel: w200 -> [_ w211]
              tunnel: w199 -> [_ w210]
              tunnel: w198 -> [_ w209]
              frame False {
              }
              frame True {
                w206 = FALSE ("Spinning")
                w216 = T3 3 items=["no dialog", "OK message", "continue or stop message", "OK message + warnings", "continue/stop + warnings"] ("type of dialog (OK msg:1)")
                n67 = property on="Synced Trigger?" class="Bool (strict)"() -> ("Value"=w208:bool)  [unwired: 2 in, 2 out]
                n68 = case shown="True" w208 {
                  tunnel: w211 -> [_ w226]
                  tunnel: w210 -> [_ w225]
                  tunnel: w209 -> [w217 w224]
                  tunnel: [w217 w218] -> w212
                  frame False {
                  }
                  frame True {
                    n69 = call <vilib>:"DAQmx Is Task Done.vi"("task/channels in"=w226, "error in"=w224) -> ("task out"=w219:refnum<k21>, "error out"=w223:errorcluster)  [unwired: 11 in, 1 out]
                    n70 = call <vilib>:"DAQmx Is Task Done.vi"("task/channels in"=w225, "error in"=w223) -> ("task out"=w221:refnum<k21>, "error out"=w222:errorcluster)  [unwired: 11 in, 1 out]
                    n71 = call <vilib>:"DAQmx Clear Task.vi"("task in"=w221, "error in"=w222) -> ("error out"=w220:errorcluster)  [unwired: 13 in]
                    n72 = call <vilib>:"DAQmx Clear Task.vi"("task in"=w219, "error in"=w220) -> ("error out"=w218:errorcluster)  [unwired: 13 in]
                  }
                }
                n73 = property on="Quivering" class="Bool (strict)"("Value"=w206) -> ()  [unwired: 2 in, 2 out]
                n74 = call <vilib>:"DAQmx Is Task Done.vi"("task/channels in"=w207, "error in"=w212) -> ("task out"=w213:refnum<k21>, "error out"=w214:errorcluster)  [unwired: 11 in, 1 out]
                n75 = call <vilib>:"DAQmx Clear Task.vi"("task in"=w213, "error in"=w214) -> ("error out"=w215:errorcluster)  [unwired: 13 in]
                n76 = property on="Spinning" class="Bool (strict)"("Value"=w206) -> ()  [unwired: 2 in, 2 out]
                n77 = call <vilib>:"Simple Error Handler.vi"("type of dialog (OK msg:1)"=w216, "error in (no error)"=w215) -> ()  [unwired: 3 in, 5 out]
              }
            }
            n78 = property on="Direction" class="Ring (strict)"("Value"=w204) -> ()  [unwired: 2 in, 2 out]
            n79 = property on="Laser Trig 1" class="Bool (strict)"("Value"=FALSE ("Laser Trig 1")) -> ()  [unwired: 2 in, 2 out]
          }
          frame #1 {
            n80 = call-poly <vilib>:"DAQmx Create Virtual Channel.vi"("maximum value"=w227, "minimum value"=w228, "physical channels"=w231) -> ("task out"=w235:refnum<k21>, "error out"=w236:errorcluster)  [unwired: 11 in]
            n81 = call-poly <vilib>:"DAQmx Write.vi"("task/channels in"=w235, "data"=w230, "timeout"=10.0, "error in"=w236) -> ("task out"=w232:refnum<k21>, "error out"=w233:errorcluster)  [unwired: 9 in, 1 out]
            n82 = call <vilib>:"DAQmx Clear Task.vi"("task in"=w232, "error in"=w233) -> ("error out"=w229:errorcluster)  [unwired: 13 in]
          }
          frame #2 {
            w239 = 0 items=["one channel for each line", "one channel for all lines"] ("line grouping")
            w245 = T3 3 items=["no dialog", "OK message", "continue or stop message", "OK message + warnings", "continue/stop + warnings"] ("type of dialog (OK msg:1)")
            n83 = call-poly <vilib>:"DAQmx Create Virtual Channel.vi"("physical channels"=w251, "error in"=w249) -> ("task out"=w250:refnum<k21>, "error out"=w248:errorcluster)  [unwired: 12 in]
            n84 = call-poly <vilib>:"DAQmx Create Virtual Channel.vi"("lines"=w237, "line grouping"=w239) -> ("task out"=w244:refnum<k21>, "error out"=w243:errorcluster)  [unwired: 12 in]
            n85 = call-poly <vilib>:"DAQmx Read.vi"("task/channels in"=w250, "number of samples per channel"=w246, "error in"=w248) -> ("data"=w254:dbl[][], "error out"=w247:errorcluster)  [unwired: 10 in, 1 out]
            n86 = Index Array(array=w254, index (row)=0) -> (element=w252:dbl[])  [unwired: 1 in]
            n87 = call-poly <vilib>:"DAQmx Write.vi"("task/channels in"=w244, "data"=bool[] [FALSE, FALSE], "error in"=w243) -> ("task out"=w241:refnum<k21>, "error out"=w242:errorcluster)  [unwired: 10 in, 1 out]
            n88 = call-poly <vilib>:"Mean.vi"("X"=w252) -> ("mean"=→"Manual Control":dbl)  [unwired: 1 out]
            n89 = call <vilib>:"Simple Error Handler.vi"("type of dialog (OK msg:1)"=w245, "error in (no error)"=w247) -> ()  [unwired: 3 in, 5 out]
            n90 = call <vilib>:"DAQmx Clear Task.vi"("task in"=w241, "error in"=w242) -> ("error out"=w240:errorcluster)  [unwired: 13 in]
            n91 = call <vilib>:"Simple Error Handler.vi"("error in (no error)"=w240) -> ()  [unwired: 4 in, 5 out]
          }
        }
        n92 = Build Array("X", "Y", w185, w185) -> (w196:dbl[])
        n93 = property on="Focus Position?" class="Bool (strict)"("Value"=w184) -> ()  [unwired: 2 in, 2 out]
        n94 = property on="Lock Z" class="Bool (strict)"("Value"=w184) -> ()  [unwired: 2 in, 2 out]
      }
      event "2D Center Find": Value Change {
        n95 = event-data() -> ()  [unwired: 1 in, 5 out]
        n96 = flat-sequence {
          tunnel: w277 -> [w303]
          tunnel: w278 -> [w304]
          tunnel: w279 -> [w305]
          tunnel: w280 -> [w306]
          tunnel: w281 -> [w307]
          tunnel: w282 -> [w308]
          tunnel: w283 -> [w309]
          tunnel: w284 -> [w310]
          tunnel: w285 -> [w311]
          tunnel: w286 -> [w312]
          tunnel: w287 -> [w313]
          tunnel: [w313] -> w276
          tunnel: [w312] -> w275
          tunnel: [w311] -> w274
          tunnel: [w310] -> w273
          tunnel: [w309] -> w272
          tunnel: [w308] -> w271
          tunnel: [w307] -> w270
          tunnel: [w306] -> w269
          tunnel: [w305] -> w268
          tunnel: [w304] -> w267
          tunnel: [w303] -> w266
          tunnel: w265 -> [w302]
          tunnel: w264 -> [w301]
          tunnel: w262 -> [w299]
          tunnel: [w299] -> w263
          tunnel: w261 -> [w298]
          tunnel: [w298] -> w260
          tunnel: w258 -> [w297]
          tunnel: [w297] -> w259
          tunnel: w257 -> [w293]
          tunnel: w256 -> [w292]
          tunnel: w276 -> [w348]
          tunnel: w275 -> [w347]
          tunnel: w274 -> [w346]
          tunnel: w273 -> [w345]
          tunnel: w272 -> [w344]
          tunnel: w271 -> [w343]
          tunnel: w270 -> [w342]
          tunnel: w269 -> [w341]
          tunnel: w268 -> [w340]
          tunnel: w267 -> [w339]
          tunnel: w266 -> [w338]
          tunnel: w263 -> [w337]
          tunnel: w260 -> [w336]
          tunnel: w259 -> [w335]
          frame #0 {
            w300 = u16 0 items=["", "North", "East", "South", "West"] ("Direction")
            w290 = FALSE ("Focus Position?")
            n97 = property on="Spinning" class="Bool (strict)"() -> ("Value"=w296:bool)  [unwired: 2 in, 2 out]
            n98 = property on="Direction" class="Ring (strict)"("Value"=w300) -> ()  [unwired: 2 in, 2 out]
            n99 = property on="Quivering" class="Bool (strict)"() -> ("Value"=w295:bool)  [unwired: 2 in, 2 out]
            n100 = property on="Focus Position?" class="Bool (strict)"("Value"=w290) -> ()  [unwired: 2 in, 2 out]
            n101 = property on="Lock Z" class="Bool (strict)"("Value"=w290) -> ()  [unwired: 2 in, 2 out]
            n102 = Or(x=w295, y=w296) -> (x .or. y?=w294:bool)
            n103 = property on="Synced Trigger?" class="Bool (strict)"() -> ("Value"=w291:bool)  [unwired: 2 in, 2 out]
            n104 = case shown="False" w294 {
              tunnel: w302 -> [_ w316]
              tunnel: w301 -> [_ w317]
              tunnel: w293 -> [_ w319]
              tunnel: w292 -> [_ w318]
              tunnel: w291 -> [_ w315]
              frame False {
              }
              frame True {
                w314 = FALSE ("Spinning")
                w324 = T3 3 items=["no dialog", "OK message", "continue or stop message", "OK message + warnings", "continue/stop + warnings"] ("type of dialog (OK msg:1)")
                n105 = case shown="True" w315 {
                  tunnel: w319 -> [_ w334]
                  tunnel: w318 -> [_ w333]
                  tunnel: w317 -> [w325 w332]
                  tunnel: [w325 w326] -> w320
                  frame False {
                  }
                  frame True {
                    n106 = call <vilib>:"DAQmx Is Task Done.vi"("task/channels in"=w334, "error in"=w332) -> ("task out"=w327:refnum<k21>, "error out"=w331:errorcluster)  [unwired: 11 in, 1 out]
                    n107 = call <vilib>:"DAQmx Is Task Done.vi"("task/channels in"=w333, "error in"=w331) -> ("task out"=w329:refnum<k21>, "error out"=w330:errorcluster)  [unwired: 11 in, 1 out]
                    n108 = call <vilib>:"DAQmx Clear Task.vi"("task in"=w329, "error in"=w330) -> ("error out"=w328:errorcluster)  [unwired: 13 in]
                    n109 = call <vilib>:"DAQmx Clear Task.vi"("task in"=w327, "error in"=w328) -> ("error out"=w326:errorcluster)  [unwired: 13 in]
                  }
                }
                n110 = call <vilib>:"DAQmx Is Task Done.vi"("task/channels in"=w316, "error in"=w320) -> ("task out"=w321:refnum<k21>, "error out"=w322:errorcluster)  [unwired: 11 in, 1 out]
                n111 = property on="Quivering" class="Bool (strict)"("Value"=w314) -> ()  [unwired: 2 in, 2 out]
                n112 = call <vilib>:"DAQmx Clear Task.vi"("task in"=w321, "error in"=w322) -> ("error out"=w323:errorcluster)  [unwired: 13 in]
                n113 = property on="Spinning" class="Bool (strict)"("Value"=w314) -> ()  [unwired: 2 in, 2 out]
                n114 = call <vilib>:"Simple Error Handler.vi"("type of dialog (OK msg:1)"=w324, "error in (no error)"=w323) -> ()  [unwired: 3 in, 5 out]
              }
            }
          }
          frame #1 {
            n115 = for {
              N: "Centering Iterations" -> [_]
              tunnel: w348 -> [w388]
              tunnel: w347 -> [w387]
              tunnel: w346 -> [w386]
              tunnel: w345 -> [w385]
              tunnel: w344 -> [w384]
              tunnel: w343 -> [w383]
              tunnel: w342 -> [w382]
              tunnel: w341 -> [w381]
              tunnel: w340 -> [w380]
              tunnel: w339 -> [w378]
              tunnel: w338 -> [w377]
              tunnel: w337 -> [w352]
              tunnel: w336 -> [w351]
              tunnel: w335 -> [w350]
              i -> [w391]
              n116 = property on="Spin Amp \n(N-S)" class="DigNum (strict)"() -> ("Value"=w360:dbl)  [unwired: 2 in, 2 out]
              n117 = property on="Y/X ration \nW-E = C*(N-S)" class="DigNum (strict)"() -> ("Value"=w358:dbl)  [unwired: 2 in, 2 out]
              n118 = Quotient & Remainder(x=w391, y=2) -> (x-y*floor(x/y)=w389:i32)  [unwired: 1 out]
              n119 = Equal To 0?(x=w389) -> (x = 0?=w371:bool)
              n120 = case shown="True" w371 {
                tunnel: [FALSE ("Scan Galvo Selection") TRUE ("Scan Galvo Selection")] -> w376
                tunnel: [w400 w405] -> w375
                tunnel: w360 -> [w399 w403]
                tunnel: [w399 w402] -> w359
                tunnel: w358 -> [_ w404]
                frame False {
                  n121 = property on="E/W" class="Slide (strict)"() -> ("Value"=w400:dbl)  [unwired: 2 in, 2 out]
                }
                frame True {
                  n122 = property on="N/S" class="Slide (strict)"() -> ("Value"=w405:dbl)  [unwired: 2 in, 2 out]
                  n123 = Multiply(x=w403, y=w404) -> (x*y=w402:dbl)
                }
              }
              n124 = property on="Scan Galvo Selection" class="Bool (strict)"("Value"=w371) -> ()  [unwired: 2 in, 2 out]
              n125 = call "121129-1D_Galvo_scan_SubVI.vi"("Analog Input Channels"=w388, "End voltage (scanned galvo)"=w380, "Voltage (fixed galvo)"=w375, "Scan Galvo Selection"=w376, "Start voltage (scanned galvo)"=w387, "number of samples per channel"=w386, "Steps"=w385, "E/W EOM"=w351, "Galvo Hard Min Voltage"=w384, "Galvo Hard Max Voltage"=w383, "Analog Out Channels"=w382, "milliseconds to wait"=w381, "N/S EOM"=w352) -> ("Delta V spacing"=w379:dbl, "Array"=w392:dbl[][])  [unwired: 1 in]
              n126 = call "121129-1D_Center_find_SubVI.vi"("Array in"=w392, "Differential Initial Conditions"=w377, "Center exclude"=w350, "Delta V spacing"=w379, "Scan Galvo Selection"=w371, "Differential Method"=w378) -> ("Sum Graph"=w357:cluster{"Array":dbl[], "dX/dt":dbl[]}[], "Amplitude"=w369:dbl, "Offset"=w361:dbl, "left"=w373:dbl, "Right"=w372:dbl, "X Y Sensor Graph"=w374:cluster{"Array":dbl[], "Array":dbl[]}[])
              n127 = Add(x=w361, y=w359) -> (x+y=w366:dbl)
              n128 = Subtract(x=w361, y=w359) -> (x-y=w362:dbl)
              n129 = case shown="False" w371 {
                tunnel: w361 -> [w395 w398]
                tunnel: [w394 w397] -> w370
                tunnel: w369 -> [w393 w396]
                frame False {
                  w394 = u16 1 items=["East-West", "North-South"] ("Text Ring")
                  n130 = property on="X" class="Slide (strict)"("Value"=w395) -> ()  [unwired: 2 in, 2 out]
                  n131 = property on="N-S Width" class="DigNum (strict)"("Value"=w393) -> ()  [unwired: 2 in, 2 out]
                }
                frame True {
                  w397 = u16 0 items=["East-West", "North-South"] ("Text Ring")
                  n132 = property on="Y" class="Slide (strict)"("Value"=w398) -> ()  [unwired: 2 in, 2 out]
                  n133 = property on="W-E Width" class="DigNum (strict)"("Value"=w396) -> ()  [unwired: 2 in, 2 out]
                }
              }
              n134 = Build Array(w362, w362) -> (w363:dbl[])
              n135 = Build Array(w366, w366) -> (w367:dbl[])
              n136 = Build Array(0.0 ("element"), 1.0 ("element")) -> (w364:dbl[])
              n137 = property on="left" class="DigNum (strict)"("Value"=w373) -> ()  [unwired: 2 in, 2 out]
              n138 = Bundle(w363, w364) -> (w356:cluster{dbl[], dbl[]})  [unwired: 1 in]
              n139 = Bundle(w367, w364) -> (w365:cluster{dbl[], dbl[]})  [unwired: 1 in]
              n140 = property on="Offset" class="DigNum (strict)"("Value"=w361) -> ()  [unwired: 2 in, 2 out]
              n141 = Insert Into Array(array=w357, index=5, new element #1=w356, new element #2=w365) -> (w354:cluster{"Array":dbl[], "dX/dt":dbl[]}[])
              n142 = property on="Amplitude" class="DigNum (strict)"("Value"=w369) -> ()  [unwired: 2 in, 2 out]
              n143 = property on="Right" class="DigNum (strict)"("Value"=w372) -> ()  [unwired: 2 in, 2 out]
              n144 = property on="X Y Sensor" class="XYGraph (strict)"("Value"=w374) -> ()  [unwired: 2 in, 2 out]
              n145 = property on="Text Ring" class="Ring (strict)"("Value"=w370) -> ()  [unwired: 2 in, 2 out]
              n146 = property on="Sum Graph" class="XYGraph (strict)"("Value"=w354) -> ()  [unwired: 2 in, 2 out]
            }
          }
          frame #2 {
            n147 = case shown="True" "Write Y/X ration \nduring center find?" {
              frame False {
              }
              frame True {
                n148 = property on="W-E Width" class="DigNum (strict)"() -> ("Value"=w409:dbl)  [unwired: 2 in, 2 out]
                n149 = property on="N-S Width" class="DigNum (strict)"() -> ("Value"=w410:dbl)  [unwired: 2 in, 2 out]
                n150 = Divide(x=w409, y=w410) -> (x/y=w408:dbl)
                n151 = property on="Y/X ration \nW-E = C*(N-S)" class="DigNum (strict)"("Value"=w408) -> ()  [unwired: 2 in, 2 out]
              }
            }
          }
        }
        n152 = Not(x="2D Center Find") -> (.not. x?=w288:bool)
      }
      event "Spin": Value Change {
        n153 = event-data() -> ()  [unwired: 1 in, 5 out]
        n154 = flat-sequence {
          tunnel: w416 -> [w437]
          tunnel: w415 -> [w436]
          tunnel: w414 -> [w435]
          tunnel: w412 -> [w434]
          tunnel: [w489] -> w425
          tunnel: [w488] -> w424
          tunnel: w421 -> [w484]
          tunnel: "EOM spin?" -> [w476]
          tunnel: [w469] -> w418
          tunnel: [w468] -> w417
          tunnel: w413 -> [w467]
          tunnel: w411 -> [w466]
          frame #0 {
            w441 = u16 0 items=["", "North", "East", "South", "West"] ("Direction")
            n155 = property on="Spinning" class="Bool (strict)"() -> ("Value"=w439:bool)  [unwired: 2 in, 2 out]
            n156 = property on="Quivering" class="Bool (strict)"() -> ("Value"=w440:bool)  [unwired: 2 in, 2 out]
            n157 = Or(x=w440, y=w439) -> (x .or. y?=w438:bool)
            n158 = case shown="True" w438 {
              tunnel: w437 -> [_ w448]
              tunnel: w436 -> [_ w447]
              tunnel: w435 -> [_ w446]
              tunnel: w434 -> [_ w444]
              frame False {
              }
              frame True {
                w442 = FALSE ("Spinning")
                w452 = T3 3 items=["no dialog", "OK message", "continue or stop message", "OK message + warnings", "continue/stop + warnings"] ("type of dialog (OK msg:1)")
                n159 = property on="Synced Trigger?" class="Bool (strict)"() -> ("Value"=w443:bool)  [unwired: 2 in, 2 out]
                n160 = case shown="True" w443 {
                  tunnel: w447 -> [_ w462]
                  tunnel: w446 -> [_ w461]
                  tunnel: w448 -> [w453 w460]
                  tunnel: [w453 w454] -> w445
                  frame False {
                  }
                  frame True {
                    n161 = call <vilib>:"DAQmx Is Task Done.vi"("task/channels in"=w462, "error in"=w460) -> ("task out"=w455:refnum<k21>, "error out"=w459:errorcluster)  [unwired: 11 in, 1 out]
                    n162 = call <vilib>:"DAQmx Is Task Done.vi"("task/channels in"=w461, "error in"=w459) -> ("task out"=w457:refnum<k21>, "error out"=w458:errorcluster)  [unwired: 11 in, 1 out]
                    n163 = call <vilib>:"DAQmx Clear Task.vi"("task in"=w457, "error in"=w458) -> ("error out"=w456:errorcluster)  [unwired: 13 in]
                    n164 = call <vilib>:"DAQmx Clear Task.vi"("task in"=w455, "error in"=w456) -> ("error out"=w454:errorcluster)  [unwired: 13 in]
                  }
                }
                n165 = call <vilib>:"DAQmx Is Task Done.vi"("task/channels in"=w444, "error in"=w445) -> ("task out"=w449:refnum<k21>, "error out"=w450:errorcluster)  [unwired: 11 in, 1 out]
                n166 = call <vilib>:"DAQmx Clear Task.vi"("task in"=w449, "error in"=w450) -> ("error out"=w451:errorcluster)  [unwired: 13 in]
                n167 = call <vilib>:"Simple Error Handler.vi"("type of dialog (OK msg:1)"=w452, "error in (no error)"=w451) -> ()  [unwired: 3 in, 5 out]
                n168 = property on="Spin" class="Bool (strict)"("Value"=w442) -> ()  [unwired: 2 in, 2 out]
                n169 = property on="Quivering" class="Bool (strict)"("Value"=w442) -> ()  [unwired: 2 in, 2 out]
              }
            }
            n170 = property on="Direction" class="Ring (strict)"("Value"=w441) -> ()  [unwired: 2 in, 2 out]
            n171 = property on="Laser Trig 1" class="Bool (strict)"("Value"=FALSE ("Laser Trig 1")) -> ()  [unwired: 2 in, 2 out]
          }
          frame #1 {
            w479 = u16 0 items=["", "Active spin for focus lock"] ("Text Ring 2")
            w505 = 10123 items=["Finite Samples"=10178, "Continuous Samples"=10123, "Hardware Timed Single Point"=12522] ("sample mode")
            n172 = property on="N/S" class="Slide (strict)"() -> ("Value"=w486:dbl)  [unwired: 2 in, 2 out]
            n173 = call-poly <vilib>:"DAQmx Create Virtual Channel.vi"("physical channels"=w484) -> ("task out"=w503:refnum<k21>, "error out"=w497:errorcluster)  [unwired: 13 in]
            n174 = property on="Notification" class="Ring (strict)"("Value"=w479) -> ()  [unwired: 2 in, 2 out]
            n175 = property on="E/W" class="Slide (strict)"() -> ("Value"=w485:dbl)  [unwired: 2 in, 2 out]
            n176 = case shown="True" "180° Shift (s)" {
              tunnel: "Phase" -> [w537 w540]
              tunnel: [w537 w539] -> w474
              frame False {
              }
              frame True {
                n177 = Add(x=w540, y=180.0) -> (x+y=w539:dbl)
              }
            }
            n178 = Multiply(x="Spin Amp (N-S)", y="Y/X ration \nW-E = C*(N-S)") -> (x*y=w480:dbl)
            n179 = case shown="False" "180° Shift" {
              tunnel: "Phase" -> [w533 w536]
              tunnel: [w533 w535] -> w472
              frame False {
              }
              frame True {
                n180 = Add(x=w536, y=180.0) -> (x+y=w535:dbl)
              }
            }
            n181 = call "130531-spin_waveform_generate_phase_shift-SubVI.vi"("Ch. 1 Amp"="Spin Amp (N-S)", "Ch. 1 Offset"=w486, "Ch. 1 Phase"=0.0, "Ch. 2 Amp"=w480, "Ch. 2 Offset"=w485, "Ch. 2 Phase"="W-E Phase Delay", "# repeats"="# repeats", "error in (no error)"=w497, "Ch. 3 Amp"="Amplitude", "frequency"="Frequency", "Ch. 3 Offset"="Offset", "# sample"="# sample", "Ch. 3 Phase"=w474, "Splice?"="Splice?", "Ch. 4 Amp"="Amplitude", "Ch. 4 Offset"="Offset", "Ch. 4 Phase"=w472) -> ("output cluster"=→"output cluster":cluster{dbl, "# sample":i32}, "Array"=w478:waveform(dbl)[], "error out"=w501:errorcluster)  [unwired: 8 in]
            n182 = case shown="False" w476 {
              tunnel: w478 -> [w544 w545]
              tunnel: [w541 w545] -> w477
              frame False {
                n183 = Array Subset(array=w544, index=0, length=2) -> (w541:waveform(dbl)[])
              }
              frame True {
              }
            }
            "Output Waveform" <- w477
            n184 = Index Array(array=w478, index=0) -> (element=w499:waveform(dbl))
            n185 = call-poly <vilib>:"DAQmx Timing.vi"("task/channels in"=w503, "sample mode"=w505, "waveform"=w499, "error in"=w501) -> ("task out"=w504:refnum<k21>, "error out"=w502:errorcluster)  [unwired: 10 in]
            n186 = case shown="True" "Synced Trigger?" {
              tunnel: w504 -> [w515 w532]
              tunnel: w502 -> [w512 w529]
              tunnel: [w511 w523] -> w489
              tunnel: [w510 w527] -> w488
              tunnel: w477 -> [w509 w530]
              tunnel: [refnum<k21> refnum ("Digital Ref. Out") w522] -> w469
              tunnel: [refnum<k21> refnum ("Counter Ref. Out") w521] -> w468
              tunnel: w467 -> [_ w520]
              tunnel: w466 -> [_ w519]
              frame False {
                w506 = u16 5 items=["", "North", "East", "South", "West", "Spin", "Sync"] ("Direction")
                n187 = property on="Direction" class="Ring (strict)"("Value"=w506) -> ()  [unwired: 2 in, 2 out]
                n188 = call-poly <vilib>:"DAQmx Write.vi"("task/channels in"=w515, "data"=w509, "error in"=w512) -> ("task out"=w514:refnum<k21>, "error out"=w513:errorcluster)  [unwired: 10 in, 1 out]
                n189 = call <vilib>:"DAQmx Start Task.vi"("task/channels in"=w514, "error in"=w513) -> ("task out"=w511:refnum<k21>, "error out"=w510:errorcluster)  [unwired: 12 in]
              }
              frame True {
                w516 = u16 6 items=["", "North", "East", "South", "West", "Spin", "Sync"] ("Direction")
                n190 = call "130604-spin_digital_trig_sync-SubVI.vi"("Analog Ch. Reference In"=w532, "counter ch. #"=w519, "Digital Data"="Digital Data", "Digital lines"=w520, "Analog Waveform"=w530, "error in (no error)"=w529, "Cycle time"="Cycle time", "Digital Time Step"="Digital  Time Step", "CO.Pulse.Term"="CO.Pulse.Term") -> ("Digital Ref. Out"=w522:refnum<k21>, "SampClk.Rate"=→"Clock Rate":dbl, "Counter Ref. Out"=w521:refnum<k21>, "Aanlog Ch. Ref. Out"=w523:refnum<k21>, "Digital Waveform Graph"=→"Digital Waveform":digitalwaveform[], "number of samples"=→"number of samples":i32, "error out"=w527:errorcluster)  [unwired: 3 in, 1 out]
                n191 = property on="Direction" class="Ring (strict)"("Value"=w516) -> ()  [unwired: 2 in, 2 out]
              }
            }
            "Spinning" <- TRUE ("Spinning")
          }
        }
        n192 = case shown="False" "EOM spin?" {
          tunnel: w420 -> [w431 w432]
          tunnel: [w426 w432] -> w421
          frame False {
            n193 = call <vilib>:"DAQmx Unflatten Channel String.vi"("names in"=w431) -> ("names out"=w430:string[])  [unwired: 13 in, 1 out]
            n194 = Array Subset(array=w430, index=0, length=2) -> (w427:string[])
            n195 = call <vilib>:"DAQmx Flatten Channel String.vi"("names in"=w427) -> ("names out"=w426:string)  [unwired: 13 in, 1 out]
          }
          frame True {
          }
        }
        n196 = Not(x="Spin") -> (.not. x?=w422:bool)
      }
      event "Quiver": Value Change {
        n197 = event-data() -> ()  [unwired: 1 in, 5 out]
        n198 = flat-sequence {
          tunnel: w553 -> [w573]
          tunnel: w554 -> [w572]
          tunnel: w548 -> [w567]
          tunnel: w547 -> [w566]
          tunnel: [w640] -> w552
          tunnel: [w639] -> w551
          tunnel: w556 -> [w637]
          tunnel: "EOM spin? (Quiver)" -> [w633]
          tunnel: w546 -> [w596]
          frame #0 {
            w571 = u16 0 items=["", "North", "East", "South", "West"] ("Direction")
            n199 = property on="Laser Trig 1" class="Bool (strict)"("Value"=FALSE ("Laser Trig 1")) -> ()  [unwired: 2 in, 2 out]
            n200 = property on="Quivering" class="Bool (strict)"() -> ("Value"=w570:bool)  [unwired: 2 in, 2 out]
            n201 = property on="Spinning" class="Bool (strict)"() -> ("Value"=w569:bool)  [unwired: 2 in, 2 out]
            n202 = Or(x=w569, y=w570) -> (x .or. y?=w568:bool)
            n203 = case shown="True" w568 {
              tunnel: w573 -> [_ w576]
              tunnel: w572 -> [_ w578]
              tunnel: w567 -> [_ w580]
              tunnel: w566 -> [_ w579]
              frame False {
              }
              frame True {
                w574 = FALSE ("Spinning")
                w584 = T3 3 items=["no dialog", "OK message", "continue or stop message", "OK message + warnings", "continue/stop + warnings"] ("type of dialog (OK msg:1)")
                n204 = property on="Synced Trigger?" class="Bool (strict)"() -> ("Value"=w575:bool)  [unwired: 2 in, 2 out]
                n205 = case shown="True" w575 {
                  tunnel: w580 -> [_ w594]
                  tunnel: w579 -> [_ w593]
                  tunnel: w578 -> [w585 w592]
                  tunnel: [w585 w586] -> w577
                  frame False {
                  }
                  frame True {
                    n206 = call <vilib>:"DAQmx Is Task Done.vi"("task/channels in"=w594, "error in"=w592) -> ("task out"=w587:refnum<k21>, "error out"=w591:errorcluster)  [unwired: 11 in, 1 out]
                    n207 = call <vilib>:"DAQmx Is Task Done.vi"("task/channels in"=w593, "error in"=w591) -> ("task out"=w589:refnum<k21>, "error out"=w590:errorcluster)  [unwired: 11 in, 1 out]
                    n208 = call <vilib>:"DAQmx Clear Task.vi"("task in"=w589, "error in"=w590) -> ("error out"=w588:errorcluster)  [unwired: 13 in]
                    n209 = call <vilib>:"DAQmx Clear Task.vi"("task in"=w587, "error in"=w588) -> ("error out"=w586:errorcluster)  [unwired: 13 in]
                  }
                }
                n210 = call <vilib>:"DAQmx Is Task Done.vi"("task/channels in"=w576, "error in"=w577) -> ("task out"=w581:refnum<k21>, "error out"=w582:errorcluster)  [unwired: 11 in, 1 out]
                n211 = property on="Quiver" class="Bool (strict)"("Value"=w574) -> ()  [unwired: 2 in, 2 out]
                n212 = call <vilib>:"DAQmx Clear Task.vi"("task in"=w581, "error in"=w582) -> ("error out"=w583:errorcluster)  [unwired: 13 in]
                n213 = property on="Quivering" class="Bool (strict)"("Value"=w574) -> ()  [unwired: 2 in, 2 out]
                n214 = call <vilib>:"Simple Error Handler.vi"("type of dialog (OK msg:1)"=w584, "error in (no error)"=w583) -> ()  [unwired: 3 in, 5 out]
              }
            }
            n215 = property on="Direction" class="Ring (strict)"("Value"=w571) -> ()  [unwired: 2 in, 2 out]
          }
          frame #1 {
            w595 = 0 items=["one channel for each line", "one channel for all lines"] ("line grouping")
            w626 = u16 0 items=["", "Active spin for focus lock"] ("Text Ring 2")
            w652 = 10123 items=["Finite Samples"=10178, "Continuous Samples"=10123, "Hardware Timed Single Point"=12522] ("sample mode")
            n216 = property on="Y/X ration \nW-E = C*(N-S)" class="DigNum (strict)"() -> ("Value"=w618:dbl)  [unwired: 2 in, 2 out]
            n217 = property on="Frequency" class="DigNum (strict)"() -> ("Value"=w619:dbl)  [unwired: 2 in, 2 out]
            n218 = property on="Spin Amp (N-S)" class="DigNum (strict)"() -> ("Value"=w620:dbl)  [unwired: 2 in, 2 out]
            n219 = property on="X" class="Slide (strict)"() -> ("Value"=w617:dbl)  [unwired: 2 in, 2 out]
            n220 = property on="Notification" class="Ring (strict)"("Value"=w626) -> ()  [unwired: 2 in, 2 out]
            n221 = call-poly <vilib>:"DAQmx Create Virtual Channel.vi"("physical channels"=w637) -> ("task out"=w650:refnum<k21>, "error out"=w643:errorcluster)  [unwired: 13 in]
            n222 = property on="Y" class="Slide (strict)"() -> ("Value"=w616:dbl)  [unwired: 2 in, 2 out]
            n223 = property on="Amplitude" class="DigNum (strict)"() -> ("Value"=w610:dbl)  [unwired: 2 in, 2 out]
            n224 = Divide(x="Quiver full amp", y=2.0) -> (x/y=w611:dbl)
            n225 = case shown="True" "180° Shift" {
              tunnel: "Phase" -> [w665 w668]
              tunnel: [w665 w667] -> w631
              frame False {
              }
              frame True {
                n226 = Add(x=w668, y=180.0) -> (x+y=w667:dbl)
              }
            }
            n227 = Multiply(x=w620, y=w618) -> (x*y=w635:dbl)
            n228 = call-poly <vilib>:"DAQmx Create Virtual Channel.vi"("lines"=w596, "line grouping"=w595) -> ("task out"=w602:refnum<k21>, "error out"=w601:errorcluster)  [unwired: 12 in]
            n229 = Divide(x=w610, y=90.0) -> (x/y=w608:dbl)
            n230 = property on="Amplitude" class="DigNum (strict)"() -> ("Value"=w606:dbl)  [unwired: 2 in, 2 out]
            n231 = case shown="True" "180° Shift" {
              tunnel: "Phase" -> [w661 w664]
              tunnel: [w661 w663] -> w629
              frame False {
              }
              frame True {
                n232 = Add(x=w664, y=180.0) -> (x+y=w663:dbl)
              }
            }
            n233 = property on="# sample" class="DigNum (strict)"() -> ("Value"=w621:i32)  [unwired: 2 in, 2 out]
            n234 = case shown="0, Default" "Quiver Direction" {
              tunnel: [180.0 ("Ch. 1 Phase") 270.0 ("Ch. 1 Phase") 0.0 ("Ch. 1 Phase") 90.0 ("Ch. 1 Phase")] -> w615
              tunnel: [90.0 ("Ch. 1 Phase") 180.0 ("Ch. 1 Phase") 270.0 ("Ch. 1 Phase") 0.0 ("Ch. 1 Phase")] -> w614
              frame 0, Default {
              }
              frame 1 {
              }
              frame 2 {
              }
              frame 3 {
              }
            }
            n235 = Divide(x=w606, y=90.0) -> (x/y=w605:dbl)
            n236 = call-poly <vilib>:"DAQmx Write.vi"("task/channels in"=w602, "data"=bool[] [FALSE, FALSE], "error in"=w601) -> ("task out"=w599:refnum<k21>, "error out"=w600:errorcluster)  [unwired: 10 in, 1 out]
            n237 = call <vilib>:"DAQmx Clear Task.vi"("task in"=w599, "error in"=w600) -> ("error out"=w598:errorcluster)  [unwired: 13 in]
            n238 = call "130501-spin_waveform_generate_quiver-SubVI.vi"("Ch. 1 Amp"=w620, "Ch. 1 Offset"=w617, "Ch. 1 Phase"=0.0, "Ch. 2 Amp"=w635, "Ch. 2 Offset"=w616, "Ch. 2 Phase"="W-E Phase", "Quiver amplitude"=w611, "error in (no error)"=w643, "Ch. 3 Amp"=w608, "frequency"=w619, "Ch. 3 Offset"="Offset", "# sample"=w621, "Ch. 3 Phase"=w631, "quiver offset Ch. 1"=w614, "Ch. 4 Amp"=w605, "quiver offset Ch. 2"=w615, "Ch. 4 Offset"="Offset", "quiver offset Ch. 3"="quiver offset", "Ch. 4 Phase"=w629, "quiver offset Ch. 4"="quiver offset") -> ("output cluster"=w622:cluster{dbl, "# sample":i32}, "Array"=w634:waveform(dbl)[], "error out"=w646:errorcluster)  [unwired: 5 in]
            n239 = call <vilib>:"Simple Error Handler.vi"("error in (no error)"=w598) -> ()  [unwired: 4 in, 5 out]
            n240 = property on="output cluster" class="Clust (strict)"("Value"=w622) -> ()  [unwired: 2 in, 2 out]
            n241 = case shown="False" w633 {
              tunnel: w634 -> [w672 w673]
              tunnel: [w669 w673] -> w623
              frame False {
                n242 = Array Subset(array=w672, index=0, length=2) -> (w669:waveform(dbl)[])
              }
              frame True {
              }
            }
            n243 = Index Array(array=w634, index=0) -> (element=w645:waveform(dbl))
            n244 = call-poly <vilib>:"DAQmx Timing.vi"("task/channels in"=w650, "sample mode"=w652, "waveform"=w645, "error in"=w646) -> ("task out"=w651:refnum<k21>, "error out"=w647:errorcluster)  [unwired: 10 in]
            n245 = property on="Output Waveform" class="WFGraph (strict)"("Value"=w623) -> ()  [unwired: 2 in, 2 out]
            n246 = call-poly <vilib>:"DAQmx Write.vi"("task/channels in"=w651, "data"=w623, "error in"=w647) -> ("task out"=w649:refnum<k21>, "error out"=w648:errorcluster)  [unwired: 10 in, 1 out]
            n247 = call <vilib>:"DAQmx Start Task.vi"("task/channels in"=w649, "error in"=w648) -> ("task out"=w640:refnum<k21>, "error out"=w639:errorcluster)  [unwired: 12 in]
            "Quivering" <- TRUE ("Spinning")
          }
        }
        n248 = case shown="False" "EOM spin? (Quiver)" {
          tunnel: w549 -> [w563 w564]
          tunnel: [w558 w564] -> w556
          frame False {
            n249 = call <vilib>:"DAQmx Unflatten Channel String.vi"("names in"=w563) -> ("names out"=w562:string[])  [unwired: 13 in, 1 out]
            n250 = Array Subset(array=w562, index=0, length=2) -> (w559:string[])
            n251 = call <vilib>:"DAQmx Flatten Channel String.vi"("names in"=w559) -> ("names out"=w558:string)  [unwired: 13 in, 1 out]
          }
          frame True {
          }
        }
        n252 = Not(x="Quiver") -> (.not. x?=w550:bool)
      }
      event "North": Value Change {
        n253 = event-data() -> ()  [unwired: 1 in, 5 out]
        n254 = flat-sequence {
          tunnel: w683 -> [w691]
          tunnel: w677 -> [w687]
          tunnel: w676 -> [w686]
          tunnel: w675 -> [w685]
          tunnel: w681 -> [w732]
          tunnel: w680 -> [w731]
          tunnel: w682 -> [w730]
          tunnel: w674 -> [w713]
          frame #0 {
            n255 = property on="Spinning" class="Bool (strict)"() -> ("Value"=w690:bool)  [unwired: 2 in, 2 out]
            n256 = property on="Quivering" class="Bool (strict)"() -> ("Value"=w689:bool)  [unwired: 2 in, 2 out]
            n257 = Or(x=w690, y=w689) -> (x .or. y?=w688:bool)
            n258 = case shown="True" w688 {
              tunnel: w691 -> [_ w698]
              tunnel: w687 -> [_ w697]
              tunnel: w686 -> [_ w696]
              tunnel: w685 -> [_ w695]
              frame False {
              }
              frame True {
                w692 = FALSE ("Spinning")
                w702 = T3 3 items=["no dialog", "OK message", "continue or stop message", "OK message + warnings", "continue/stop + warnings"] ("type of dialog (OK msg:1)")
                n259 = property on="Synced Trigger?" class="Bool (strict)"() -> ("Value"=w693:bool)  [unwired: 2 in, 2 out]
                n260 = case shown="True" w693 {
                  tunnel: w697 -> [_ w712]
                  tunnel: w696 -> [_ w711]
                  tunnel: w695 -> [w703 w710]
                  tunnel: [w703 w704] -> w694
                  frame False {
                  }
                  frame True {
                    n261 = call <vilib>:"DAQmx Is Task Done.vi"("task/channels in"=w712, "error in"=w710) -> ("task out"=w705:refnum<k21>, "error out"=w709:errorcluster)  [unwired: 11 in, 1 out]
                    n262 = call <vilib>:"DAQmx Is Task Done.vi"("task/channels in"=w711, "error in"=w709) -> ("task out"=w707:refnum<k21>, "error out"=w708:errorcluster)  [unwired: 11 in, 1 out]
                    n263 = call <vilib>:"DAQmx Clear Task.vi"("task in"=w707, "error in"=w708) -> ("error out"=w706:errorcluster)  [unwired: 13 in]
                    n264 = call <vilib>:"DAQmx Clear Task.vi"("task in"=w705, "error in"=w706) -> ("error out"=w704:errorcluster)  [unwired: 13 in]
                  }
                }
                n265 = property on="Spinning" class="Bool (strict)"("Value"=w692) -> ()  [unwired: 2 in, 2 out]
                n266 = property on="Quivering" class="Bool (strict)"("Value"=w692) -> ()  [unwired: 2 in, 2 out]
                n267 = call <vilib>:"DAQmx Is Task Done.vi"("task/channels in"=w698, "error in"=w694) -> ("task out"=w699:refnum<k21>, "error out"=w700:errorcluster)  [unwired: 11 in, 1 out]
                n268 = call <vilib>:"DAQmx Clear Task.vi"("task in"=w699, "error in"=w700) -> ("error out"=w701:errorcluster)  [unwired: 13 in]
                n269 = call <vilib>:"Simple Error Handler.vi"("type of dialog (OK msg:1)"=w702, "error in (no error)"=w701) -> ()  [unwired: 3 in, 5 out]
              }
            }
            n270 = property on="Laser Trig 1" class="Bool (strict)"("Value"=FALSE ("Laser Trig 1")) -> ()  [unwired: 2 in, 2 out]
          }
          frame #1 {
            w714 = 0 items=["one channel for each line", "one channel for all lines"] ("line grouping")
            w722 = u16 1 items=["", "North", "East", "South", "West"] ("Direction")
            w727 = T3 3 items=["no dialog", "OK message", "continue or stop message", "OK message + warnings", "continue/stop + warnings"] ("type of dialog (OK msg:1)")
            n271 = property on="X" class="Slide (strict)"() -> ("Value"=w726:dbl)  [unwired: 2 in, 2 out]
            n272 = property on="Y" class="Slide (strict)"() -> ("Value"=w723:dbl)  [unwired: 2 in, 2 out]
            n273 = property on="Spin Amp (N-S)" class="DigNum (strict)"() -> ("Value"=w725:dbl)  [unwired: 2 in, 2 out]
            n274 = property on="Direction" class="Ring (strict)"("Value"=w722) -> ()  [unwired: 2 in, 2 out]
            n275 = Add(x=w726, y=w725) -> (x+y=w724:dbl)
            n276 = call-poly <vilib>:"DAQmx Create Virtual Channel.vi"("lines"=w713, "line grouping"=w714) -> ("task out"=w720:refnum<k21>, "error out"=w719:errorcluster)  [unwired: 12 in]
            n277 = property on="EOM Voltage (Ch. 3)" class="Slide (strict)"() -> ("Value"=w721:dbl)  [unwired: 2 in, 2 out]
            n278 = call-poly <vilib>:"DAQmx Create Virtual Channel.vi"("maximum value"=w732, "minimum value"=w731, "physical channels"=w730) -> ("task out"=w737:refnum<k21>, "error out"=w738:errorcluster)  [unwired: 11 in]
            n279 = Build Array(w724, w723, w721, 0.0 ("element")) -> (w733:dbl[])
            n280 = call-poly <vilib>:"DAQmx Write.vi"("task/channels in"=w720, "data"=bool[] [FALSE, FALSE], "error in"=w719) -> ("task out"=w717:refnum<k21>, "error out"=w718:errorcluster)  [unwired: 10 in, 1 out]
            n281 = call-poly <vilib>:"DAQmx Write.vi"("task/channels in"=w737, "data"=w733, "timeout"=10.0, "error in"=w738) -> ("task out"=w734:refnum<k21>, "error out"=w735:errorcluster)  [unwired: 9 in, 1 out]
            n282 = call <vilib>:"DAQmx Clear Task.vi"("task in"=w717, "error in"=w718) -> ("error out"=w716:errorcluster)  [unwired: 13 in]
            n283 = call <vilib>:"Simple Error Handler.vi"("error in (no error)"=w716) -> ()  [unwired: 4 in, 5 out]
            n284 = call <vilib>:"DAQmx Clear Task.vi"("task in"=w734, "error in"=w735) -> ("error out"=w728:errorcluster)  [unwired: 13 in]
            n285 = call <vilib>:"Simple Error Handler.vi"("type of dialog (OK msg:1)"=w727, "error in (no error)"=w728) -> ()  [unwired: 3 in, 5 out]
          }
        }
        n286 = Not(x="North") -> (.not. x?=w678:bool)
      }
      event "East": Value Change {
        n287 = event-data() -> ()  [unwired: 1 in, 5 out]
        n288 = flat-sequence {
          tunnel: [w756] -> _
          tunnel: w748 -> [w756]
          tunnel: w742 -> [w752]
          tunnel: w741 -> [w751]
          tunnel: w740 -> [w750]
          tunnel: w746 -> [w799]
          tunnel: w747 -> [w798]
          tunnel: w745 -> [w797]
          tunnel: w739 -> [w778]
          frame #0 {
            n289 = property on="Quivering" class="Bool (strict)"() -> ("Value"=w755:bool)  [unwired: 2 in, 2 out]
            n290 = property on="Spinning" class="Bool (strict)"() -> ("Value"=w754:bool)  [unwired: 2 in, 2 out]
            n291 = Or(x=w754, y=w755) -> (x .or. y?=w753:bool)
            n292 = case shown="True" w753 {
              tunnel: w756 -> [_ w763]
              tunnel: w752 -> [_ w762]
              tunnel: w751 -> [_ w761]
              tunnel: w750 -> [_ w760]
              frame False {
              }
              frame True {
                w757 = FALSE ("Spinning")
                w767 = T3 3 items=["no dialog", "OK message", "continue or stop message", "OK message + warnings", "continue/stop + warnings"] ("type of dialog (OK msg:1)")
                n293 = property on="Synced Trigger?" class="Bool (strict)"() -> ("Value"=w758:bool)  [unwired: 2 in, 2 out]
                n294 = case shown="True" w758 {
                  tunnel: w762 -> [_ w777]
                  tunnel: w761 -> [_ w776]
                  tunnel: w760 -> [w768 w775]
                  tunnel: [w768 w769] -> w759
                  frame False {
                  }
                  frame True {
                    n295 = call <vilib>:"DAQmx Is Task Done.vi"("task/channels in"=w777, "error in"=w775) -> ("task out"=w770:refnum<k21>, "error out"=w774:errorcluster)  [unwired: 11 in, 1 out]
                    n296 = call <vilib>:"DAQmx Is Task Done.vi"("task/channels in"=w776, "error in"=w774) -> ("task out"=w772:refnum<k21>, "error out"=w773:errorcluster)  [unwired: 11 in, 1 out]
                    n297 = call <vilib>:"DAQmx Clear Task.vi"("task in"=w772, "error in"=w773) -> ("error out"=w771:errorcluster)  [unwired: 13 in]
                    n298 = call <vilib>:"DAQmx Clear Task.vi"("task in"=w770, "error in"=w771) -> ("error out"=w769:errorcluster)  [unwired: 13 in]
                  }
                }
                n299 = property on="Spinning" class="Bool (strict)"("Value"=w757) -> ()  [unwired: 2 in, 2 out]
                n300 = property on="Quivering" class="Bool (strict)"("Value"=w757) -> ()  [unwired: 2 in, 2 out]
                n301 = call <vilib>:"DAQmx Is Task Done.vi"("task/channels in"=w763, "error in"=w759) -> ("task out"=w764:refnum<k21>, "error out"=w765:errorcluster)  [unwired: 11 in, 1 out]
                n302 = call <vilib>:"DAQmx Clear Task.vi"("task in"=w764, "error in"=w765) -> ("error out"=w766:errorcluster)  [unwired: 13 in]
                n303 = call <vilib>:"Simple Error Handler.vi"("type of dialog (OK msg:1)"=w767, "error in (no error)"=w766) -> ()  [unwired: 3 in, 5 out]
              }
            }
            n304 = property on="Laser Trig 1" class="Bool (strict)"("Value"=FALSE ("Laser Trig 1")) -> ()  [unwired: 2 in, 2 out]
          }
          frame #1 {
            w779 = 0 items=["one channel for each line", "one channel for all lines"] ("line grouping")
            w787 = u16 2 items=["", "North", "East", "South", "West"] ("Direction")
            w794 = T3 3 items=["no dialog", "OK message", "continue or stop message", "OK message + warnings", "continue/stop + warnings"] ("type of dialog (OK msg:1)")
            n305 = property on="X" class="Slide (strict)"() -> ("Value"=w793:dbl)  [unwired: 2 in, 2 out]
            n306 = property on="Y" class="Slide (strict)"() -> ("Value"=w790:dbl)  [unwired: 2 in, 2 out]
            n307 = property on="Spin Amp (N-S)" class="DigNum (strict)"() -> ("Value"=w789:dbl)  [unwired: 2 in, 2 out]
            n308 = property on="Y/X ration \nW-E = C*(N-S)" class="DigNum (strict)"() -> ("Value"=w791:dbl)  [unwired: 2 in, 2 out]
            n309 = Multiply(x=w789, y=w791) -> (x*y=w788:dbl)
            n310 = Subtract(x=w790, y=w788) -> (x-y=w792:dbl)
            n311 = call-poly <vilib>:"DAQmx Create Virtual Channel.vi"("lines"=w778, "line grouping"=w779) -> ("task out"=w785:refnum<k21>, "error out"=w784:errorcluster)  [unwired: 12 in]
            n312 = property on="EOM Voltage (Ch. 3)" class="Slide (strict)"() -> ("Value"=w786:dbl)  [unwired: 2 in, 2 out]
            n313 = call-poly <vilib>:"DAQmx Create Virtual Channel.vi"("maximum value"=w799, "minimum value"=w798, "physical channels"=w797) -> ("task out"=w804:refnum<k21>, "error out"=w805:errorcluster)  [unwired: 11 in]
            n314 = Build Array(w793, w792, w786, 0.0 ("element")) -> (w800:dbl[])
            n315 = call-poly <vilib>:"DAQmx Write.vi"("task/channels in"=w785, "data"=bool[] [FALSE, FALSE], "error in"=w784) -> ("task out"=w782:refnum<k21>, "error out"=w783:errorcluster)  [unwired: 10 in, 1 out]
            n316 = call-poly <vilib>:"DAQmx Write.vi"("task/channels in"=w804, "data"=w800, "timeout"=10.0, "error in"=w805) -> ("task out"=w801:refnum<k21>, "error out"=w802:errorcluster)  [unwired: 9 in, 1 out]
            n317 = call <vilib>:"DAQmx Clear Task.vi"("task in"=w782, "error in"=w783) -> ("error out"=w781:errorcluster)  [unwired: 13 in]
            n318 = call <vilib>:"Simple Error Handler.vi"("error in (no error)"=w781) -> ()  [unwired: 4 in, 5 out]
            n319 = call <vilib>:"DAQmx Clear Task.vi"("task in"=w801, "error in"=w802) -> ("error out"=w795:errorcluster)  [unwired: 13 in]
            n320 = property on="Direction" class="Ring (strict)"("Value"=w787) -> ()  [unwired: 2 in, 2 out]
            n321 = call <vilib>:"Simple Error Handler.vi"("type of dialog (OK msg:1)"=w794, "error in (no error)"=w795) -> ()  [unwired: 3 in, 5 out]
          }
        }
        n322 = Not(x="East") -> (.not. x?=w744:bool)
      }
      event "South": Value Change {
        n323 = event-data() -> ()  [unwired: 1 in, 5 out]
        n324 = flat-sequence {
          tunnel: w815 -> [w823]
          tunnel: w814 -> [w822]
          tunnel: w807 -> [w818]
          tunnel: w806 -> [w817]
          tunnel: w812 -> [w864]
          tunnel: w813 -> [w863]
          tunnel: w811 -> [w862]
          tunnel: w808 -> [w845]
          frame #0 {
            n325 = property on="Spinning" class="Bool (strict)"() -> ("Value"=w820:bool)  [unwired: 2 in, 2 out]
            n326 = property on="Quivering" class="Bool (strict)"() -> ("Value"=w821:bool)  [unwired: 2 in, 2 out]
            n327 = Or(x=w820, y=w821) -> (x .or. y?=w819:bool)
            n328 = case shown="True" w819 {
              tunnel: w823 -> [_ w826]
              tunnel: w822 -> [_ w827]
              tunnel: w818 -> [_ w829]
              tunnel: w817 -> [_ w828]
              frame False {
              }
              frame True {
                w824 = FALSE ("Spinning")
                w834 = T3 3 items=["no dialog", "OK message", "continue or stop message", "OK message + warnings", "continue/stop + warnings"] ("type of dialog (OK msg:1)")
                n329 = property on="Synced Trigger?" class="Bool (strict)"() -> ("Value"=w825:bool)  [unwired: 2 in, 2 out]
                n330 = case shown="True" w825 {
                  tunnel: w829 -> [_ w844]
                  tunnel: w828 -> [_ w843]
                  tunnel: w827 -> [w835 w842]
                  tunnel: [w835 w836] -> w830
                  frame False {
                  }
                  frame True {
                    n331 = call <vilib>:"DAQmx Is Task Done.vi"("task/channels in"=w844, "error in"=w842) -> ("task out"=w837:refnum<k21>, "error out"=w841:errorcluster)  [unwired: 11 in, 1 out]
                    n332 = call <vilib>:"DAQmx Is Task Done.vi"("task/channels in"=w843, "error in"=w841) -> ("task out"=w839:refnum<k21>, "error out"=w840:errorcluster)  [unwired: 11 in, 1 out]
                    n333 = call <vilib>:"DAQmx Clear Task.vi"("task in"=w839, "error in"=w840) -> ("error out"=w838:errorcluster)  [unwired: 13 in]
                    n334 = call <vilib>:"DAQmx Clear Task.vi"("task in"=w837, "error in"=w838) -> ("error out"=w836:errorcluster)  [unwired: 13 in]
                  }
                }
                n335 = call <vilib>:"DAQmx Is Task Done.vi"("task/channels in"=w826, "error in"=w830) -> ("task out"=w831:refnum<k21>, "error out"=w832:errorcluster)  [unwired: 11 in, 1 out]
                n336 = call <vilib>:"DAQmx Clear Task.vi"("task in"=w831, "error in"=w832) -> ("error out"=w833:errorcluster)  [unwired: 13 in]
                n337 = property on="Spinning" class="Bool (strict)"("Value"=w824) -> ()  [unwired: 2 in, 2 out]
                n338 = property on="Quivering" class="Bool (strict)"("Value"=w824) -> ()  [unwired: 2 in, 2 out]
                n339 = call <vilib>:"Simple Error Handler.vi"("type of dialog (OK msg:1)"=w834, "error in (no error)"=w833) -> ()  [unwired: 3 in, 5 out]
              }
            }
            n340 = property on="Laser Trig 1" class="Bool (strict)"("Value"=FALSE ("Laser Trig 1")) -> ()  [unwired: 2 in, 2 out]
          }
          frame #1 {
            w846 = 0 items=["one channel for each line", "one channel for all lines"] ("line grouping")
            w854 = u16 3 items=["", "North", "East", "South", "West"] ("Direction")
            w859 = T3 3 items=["no dialog", "OK message", "continue or stop message", "OK message + warnings", "continue/stop + warnings"] ("type of dialog (OK msg:1)")
            n341 = property on="X" class="Slide (strict)"() -> ("Value"=w855:dbl)  [unwired: 2 in, 2 out]
            n342 = property on="Y" class="Slide (strict)"() -> ("Value"=w857:dbl)  [unwired: 2 in, 2 out]
            n343 = property on="Spin Amp (N-S)" class="DigNum (strict)"() -> ("Value"=w856:dbl)  [unwired: 2 in, 2 out]
            n344 = property on="Direction" class="Ring (strict)"("Value"=w854) -> ()  [unwired: 2 in, 2 out]
            n345 = Subtract(x=w855, y=w856) -> (x-y=w858:dbl)
            n346 = call-poly <vilib>:"DAQmx Create Virtual Channel.vi"("lines"=w845, "line grouping"=w846) -> ("task out"=w852:refnum<k21>, "error out"=w851:errorcluster)  [unwired: 12 in]
            n347 = property on="EOM Voltage (Ch. 3)" class="Slide (strict)"() -> ("Value"=w853:dbl)  [unwired: 2 in, 2 out]
            n348 = call-poly <vilib>:"DAQmx Create Virtual Channel.vi"("maximum value"=w864, "minimum value"=w863, "physical channels"=w862) -> ("task out"=w869:refnum<k21>, "error out"=w870:errorcluster)  [unwired: 11 in]
            n349 = Build Array(w858, w857, w853, 0.0 ("element")) -> (w865:dbl[])
            n350 = call-poly <vilib>:"DAQmx Write.vi"("task/channels in"=w852, "data"=bool[] [FALSE, FALSE], "error in"=w851) -> ("task out"=w849:refnum<k21>, "error out"=w850:errorcluster)  [unwired: 10 in, 1 out]
            n351 = call-poly <vilib>:"DAQmx Write.vi"("task/channels in"=w869, "data"=w865, "timeout"=10.0, "error in"=w870) -> ("task out"=w866:refnum<k21>, "error out"=w867:errorcluster)  [unwired: 9 in, 1 out]
            n352 = call <vilib>:"DAQmx Clear Task.vi"("task in"=w849, "error in"=w850) -> ("error out"=w848:errorcluster)  [unwired: 13 in]
            n353 = call <vilib>:"DAQmx Clear Task.vi"("task in"=w866, "error in"=w867) -> ("error out"=w860:errorcluster)  [unwired: 13 in]
            n354 = call <vilib>:"Simple Error Handler.vi"("error in (no error)"=w848) -> ()  [unwired: 4 in, 5 out]
            n355 = call <vilib>:"Simple Error Handler.vi"("type of dialog (OK msg:1)"=w859, "error in (no error)"=w860) -> ()  [unwired: 3 in, 5 out]
          }
        }
        n356 = Not(x="South") -> (.not. x?=w809:bool)
      }
      event "West": Value Change {
        n357 = event-data() -> ()  [unwired: 1 in, 5 out]
        n358 = flat-sequence {
          tunnel: w880 -> [w888]
          tunnel: w879 -> [w884]
          tunnel: w872 -> [w883]
          tunnel: w871 -> [w882]
          tunnel: w877 -> [w931]
          tunnel: w878 -> [w930]
          tunnel: w876 -> [w929]
          tunnel: w873 -> [w910]
          frame #0 {
            n359 = property on="Spinning" class="Bool (strict)"() -> ("Value"=w886:bool)  [unwired: 2 in, 2 out]
            n360 = property on="Quivering" class="Bool (strict)"() -> ("Value"=w887:bool)  [unwired: 2 in, 2 out]
            n361 = Or(x=w886, y=w887) -> (x .or. y?=w885:bool)
            n362 = case shown="True" w885 {
              tunnel: w888 -> [_ w895]
              tunnel: w884 -> [_ w894]
              tunnel: w883 -> [_ w892]
              tunnel: w882 -> [_ w891]
              frame False {
              }
              frame True {
                w889 = FALSE ("Spinning")
                w899 = T3 3 items=["no dialog", "OK message", "continue or stop message", "OK message + warnings", "continue/stop + warnings"] ("type of dialog (OK msg:1)")
                n363 = property on="Synced Trigger?" class="Bool (strict)"() -> ("Value"=w890:bool)  [unwired: 2 in, 2 out]
                n364 = case shown="True" w890 {
                  tunnel: w892 -> [_ w909]
                  tunnel: w891 -> [_ w908]
                  tunnel: w894 -> [w900 w907]
                  tunnel: [w900 w901] -> w893
                  frame False {
                  }
                  frame True {
                    n365 = call <vilib>:"DAQmx Is Task Done.vi"("task/channels in"=w909, "error in"=w907) -> ("task out"=w902:refnum<k21>, "error out"=w906:errorcluster)  [unwired: 11 in, 1 out]
                    n366 = call <vilib>:"DAQmx Is Task Done.vi"("task/channels in"=w908, "error in"=w906) -> ("task out"=w904:refnum<k21>, "error out"=w905:errorcluster)  [unwired: 11 in, 1 out]
                    n367 = call <vilib>:"DAQmx Clear Task.vi"("task in"=w904, "error in"=w905) -> ("error out"=w903:errorcluster)  [unwired: 13 in]
                    n368 = call <vilib>:"DAQmx Clear Task.vi"("task in"=w902, "error in"=w903) -> ("error out"=w901:errorcluster)  [unwired: 13 in]
                  }
                }
                n369 = call <vilib>:"DAQmx Is Task Done.vi"("task/channels in"=w895, "error in"=w893) -> ("task out"=w896:refnum<k21>, "error out"=w897:errorcluster)  [unwired: 11 in, 1 out]
                n370 = call <vilib>:"DAQmx Clear Task.vi"("task in"=w896, "error in"=w897) -> ("error out"=w898:errorcluster)  [unwired: 13 in]
                n371 = property on="Spinning" class="Bool (strict)"("Value"=w889) -> ()  [unwired: 2 in, 2 out]
                n372 = property on="Quivering" class="Bool (strict)"("Value"=w889) -> ()  [unwired: 2 in, 2 out]
                n373 = call <vilib>:"Simple Error Handler.vi"("type of dialog (OK msg:1)"=w899, "error in (no error)"=w898) -> ()  [unwired: 3 in, 5 out]
              }
            }
            n374 = property on="Laser Trig 1" class="Bool (strict)"("Value"=FALSE ("Laser Trig 1")) -> ()  [unwired: 2 in, 2 out]
          }
          frame #1 {
            w911 = 0 items=["one channel for each line", "one channel for all lines"] ("line grouping")
            w919 = u16 4 items=["", "North", "East", "South", "West"] ("Direction")
            w926 = T3 3 items=["no dialog", "OK message", "continue or stop message", "OK message + warnings", "continue/stop + warnings"] ("type of dialog (OK msg:1)")
            n375 = property on="X" class="Slide (strict)"() -> ("Value"=w925:dbl)  [unwired: 2 in, 2 out]
            n376 = property on="Y" class="Slide (strict)"() -> ("Value"=w923:dbl)  [unwired: 2 in, 2 out]
            n377 = property on="Spin Amp (N-S)" class="DigNum (strict)"() -> ("Value"=w922:dbl)  [unwired: 2 in, 2 out]
            n378 = property on="Y/X ration \nW-E = C*(N-S)" class="DigNum (strict)"() -> ("Value"=w921:dbl)  [unwired: 2 in, 2 out]
            n379 = Multiply(x=w922, y=w921) -> (x*y=w920:dbl)
            n380 = Add(x=w923, y=w920) -> (x+y=w924:dbl)
            n381 = call-poly <vilib>:"DAQmx Create Virtual Channel.vi"("lines"=w910, "line grouping"=w911) -> ("task out"=w917:refnum<k21>, "error out"=w916:errorcluster)  [unwired: 12 in]
            n382 = property on="EOM Voltage (Ch. 3)" class="Slide (strict)"() -> ("Value"=w918:dbl)  [unwired: 2 in, 2 out]
            n383 = call-poly <vilib>:"DAQmx Create Virtual Channel.vi"("maximum value"=w931, "minimum value"=w930, "physical channels"=w929) -> ("task out"=w936:refnum<k21>, "error out"=w937:errorcluster)  [unwired: 11 in]
            n384 = Build Array(w925, w924, w918, 0.0 ("element")) -> (w932:dbl[])
            n385 = call-poly <vilib>:"DAQmx Write.vi"("task/channels in"=w917, "data"=bool[] [FALSE, FALSE], "error in"=w916) -> ("task out"=w914:refnum<k21>, "error out"=w915:errorcluster)  [unwired: 10 in, 1 out]
            n386 = call-poly <vilib>:"DAQmx Write.vi"("task/channels in"=w936, "data"=w932, "timeout"=10.0, "error in"=w937) -> ("task out"=w933:refnum<k21>, "error out"=w934:errorcluster)  [unwired: 9 in, 1 out]
            n387 = call <vilib>:"DAQmx Clear Task.vi"("task in"=w914, "error in"=w915) -> ("error out"=w913:errorcluster)  [unwired: 13 in]
            n388 = call <vilib>:"Simple Error Handler.vi"("error in (no error)"=w913) -> ()  [unwired: 4 in, 5 out]
            n389 = call <vilib>:"DAQmx Clear Task.vi"("task in"=w933, "error in"=w934) -> ("error out"=w927:errorcluster)  [unwired: 13 in]
            n390 = property on="Direction" class="Ring (strict)"("Value"=w919) -> ()  [unwired: 2 in, 2 out]
            n391 = call <vilib>:"Simple Error Handler.vi"("type of dialog (OK msg:1)"=w926, "error in (no error)"=w927) -> ()  [unwired: 3 in, 5 out]
          }
        }
        n392 = Not(x="West") -> (.not. x?=w875:bool)
      }
      event "EOM Voltage (Ch. 3)": Value Change {
        n393 = event-data() -> ()  [unwired: 1 in, 5 out]
        n394 = property on="EOM spin?" class="Bool (strict)"() -> ("Value"=w940:bool)  [unwired: 2 in, 2 out]
        n395 = case shown="False" w940 {
          tunnel: w941 -> [w945 _]
          frame False {
            w953 = T3 3 items=["no dialog", "OK message", "continue or stop message", "OK message + warnings", "continue/stop + warnings"] ("type of dialog (OK msg:1)")
            n396 = call <vilib>:"DAQmx Unflatten Channel String.vi"("names in"=w945) -> ("names out"=w949:string[])  [unwired: 13 in, 1 out]
            n397 = Array Subset(array=w949, index=2, length=1) -> (w946:string[])
            n398 = call <vilib>:"DAQmx Flatten Channel String.vi"("names in"=w946) -> ("names out"=w944:string)  [unwired: 13 in, 1 out]
            n399 = call-poly <vilib>:"DAQmx Create Virtual Channel.vi"("maximum value"=1.0, "minimum value"=-1.0, "physical channels"=w944) -> ("task out"=w958:refnum<k21>, "error out"=w959:errorcluster)  [unwired: 11 in]
            n400 = call-poly <vilib>:"DAQmx Write.vi"("task/channels in"=w958, "data"="EOM Voltage (Ch. 3)", "timeout"=10.0, "error in"=w959) -> ("task out"=w955:refnum<k21>, "error out"=w956:errorcluster)  [unwired: 9 in, 1 out]
            n401 = call <vilib>:"DAQmx Clear Task.vi"("task in"=w955, "error in"=w956) -> ("error out"=w954:errorcluster)  [unwired: 13 in]
            n402 = call <vilib>:"Simple Error Handler.vi"("type of dialog (OK msg:1)"=w953, "error in (no error)"=w954) -> ()  [unwired: 3 in, 5 out]
          }
          frame True {
            w960 = u16 3 items=["", "Spin must be activated for focus lock", "Spin must be activated for focus detection", "Disable EOM spin"] ("Notification")
            n403 = property on="Notification" class="Ring (strict)"("Value"=w960) -> ()  [unwired: 2 in, 2 out]
          }
        }
      }
      event "Laser Trig 1": Value Change {
        w966 = 0 items=["one channel for each line", "one channel for all lines"] ("line grouping")
        n404 = event-data() -> ()  [unwired: 1 in, 5 out]
        n405 = property on="Synced Trigger?" class="Bool (strict)"() -> ("Value"=w970:bool)  [unwired: 2 in, 2 out]
        n406 = case shown="True" w970 {
          tunnel: w972 -> [_ w986]
          tunnel: w971 -> [_ w985]
          tunnel: w969 -> [w977 w984]
          tunnel: [w977 w978] -> w968
          frame False {
          }
          frame True {
            n407 = call <vilib>:"DAQmx Is Task Done.vi"("task/channels in"=w986, "error in"=w984) -> ("task out"=w979:refnum<k21>, "error out"=w983:errorcluster)  [unwired: 11 in, 1 out]
            n408 = call <vilib>:"DAQmx Is Task Done.vi"("task/channels in"=w985, "error in"=w983) -> ("task out"=w981:refnum<k21>, "error out"=w982:errorcluster)  [unwired: 11 in, 1 out]
            n409 = call <vilib>:"DAQmx Clear Task.vi"("task in"=w981, "error in"=w982) -> ("error out"=w980:errorcluster)  [unwired: 13 in]
            n410 = call <vilib>:"DAQmx Clear Task.vi"("task in"=w979, "error in"=w980) -> ("error out"=w978:errorcluster)  [unwired: 13 in]
          }
        }
        n411 = call-poly <vilib>:"DAQmx Create Virtual Channel.vi"("lines"=w967, "line grouping"=w966) -> ("task out"=w963:refnum<k21>, "error out"=w975:errorcluster)  [unwired: 12 in]
        n412 = Build Array(FALSE ("Boolean"), "Laser Trig 1") -> (w964:bool[])
        n413 = call-poly <vilib>:"DAQmx Write.vi"("task/channels in"=w963, "data"=w964, "error in"=w975) -> ("task out"=w962:refnum<k21>, "error out"=w974:errorcluster)  [unwired: 10 in, 1 out]
        n414 = call <vilib>:"DAQmx Clear Task.vi"("task in"=w962, "error in"=w974) -> ("error out"=w973:errorcluster)  [unwired: 13 in]
        n415 = call <vilib>:"Simple Error Handler.vi"("error in (no error)"=w973) -> ()  [unwired: 4 in, 5 out]
      }
      event "Stop spin", "Center", "EOM spin?", "180° Shift (s)", "180° Shift": Value Change {
        w991 = u16 0 items=["", "Spin must be activated for focus lock", "Spin must be activated for focus detection", "Disable EOM spin"] ("Notification")
        w994 = FALSE ("Focus Position?")
        n416 = event-data() -> ()  [unwired: 1 in, 5 out]
        n417 = flat-sequence {
          tunnel: w998 -> [w1007]
          tunnel: w990 -> [w1003]
          tunnel: w989 -> [w1002]
          tunnel: w988 -> [w1001]
          tunnel: w997 -> [w1044]
          tunnel: w996 -> [w1043]
          tunnel: w995 -> [w1042]
          tunnel: w987 -> [w1036]
          frame #0 {
            n418 = property on="Synced Trigger?" class="Bool (strict)"() -> ("Value"=w1000:bool)  [unwired: 2 in, 2 out]
            n419 = property on="Spinning" class="Bool (strict)"() -> ("Value"=w1006:bool)  [unwired: 2 in, 2 out]
            n420 = property on="Quivering" class="Bool (strict)"() -> ("Value"=w1004:bool)  [unwired: 2 in, 2 out]
            n421 = Or(x=w1006, y=w1004) -> (x .or. y?=w1005:bool)
            n422 = case shown="True" w1005 {
              tunnel: w1007 -> [_ w1014]
              tunnel: w1003 -> [_ w1012]
              tunnel: w1002 -> [_ w1011]
              tunnel: w1001 -> [_ w1010]
              tunnel: w1000 -> [_ w1009]
              frame False {
              }
              frame True {
                w1013 = FALSE ("Spinning")
                w1018 = T3 3 items=["no dialog", "OK message", "continue or stop message", "OK message + warnings", "continue/stop + warnings"] ("type of dialog (OK msg:1)")
                n423 = case shown="True" w1009 {
                  tunnel: w1012 -> [_ w1028]
                  tunnel: w1011 -> [_ w1027]
                  tunnel: w1010 -> [w1019 w1026]
                  tunnel: [w1019 w1020] -> w1008
                  frame False {
                  }
                  frame True {
                    n424 = call <vilib>:"DAQmx Is Task Done.vi"("task/channels in"=w1028, "error in"=w1026) -> ("task out"=w1021:refnum<k21>, "error out"=w1025:errorcluster)  [unwired: 11 in, 1 out]
                    n425 = call <vilib>:"DAQmx Is Task Done.vi"("task/channels in"=w1027, "error in"=w1025) -> ("task out"=w1023:refnum<k21>, "error out"=w1024:errorcluster)  [unwired: 11 in, 1 out]
                    n426 = call <vilib>:"DAQmx Clear Task.vi"("task in"=w1023, "error in"=w1024) -> ("error out"=w1022:errorcluster)  [unwired: 13 in]
                    n427 = call <vilib>:"DAQmx Clear Task.vi"("task in"=w1021, "error in"=w1022) -> ("error out"=w1020:errorcluster)  [unwired: 13 in]
                  }
                }
                n428 = property on="Spinning" class="Bool (strict)"("Value"=w1013) -> ()  [unwired: 2 in, 2 out]
                n429 = property on="Quivering" class="Bool (strict)"("Value"=w1013) -> ()  [unwired: 2 in, 2 out]
                n430 = call <vilib>:"DAQmx Is Task Done.vi"("task/channels in"=w1014, "error in"=w1008) -> ("task out"=w1015:refnum<k21>, "error out"=w1016:errorcluster)  [unwired: 11 in, 1 out]
                n431 = call <vilib>:"DAQmx Clear Task.vi"("task in"=w1015, "error in"=w1016) -> ("error out"=w1017:errorcluster)  [unwired: 13 in]
                n432 = call <vilib>:"Simple Error Handler.vi"("type of dialog (OK msg:1)"=w1018, "error in (no error)"=w1017) -> ()  [unwired: 3 in, 5 out]
              }
            }
            n433 = property on="Laser Trig 1" class="Bool (strict)"("Value"=FALSE ("Laser Trig 1")) -> ()  [unwired: 2 in, 2 out]
          }
          frame #1 {
            w1030 = 0 items=["one channel for each line", "one channel for all lines"] ("line grouping")
            w1038 = u16 0 items=["", "North", "East", "South", "West"] ("Notification 2")
            w1039 = T3 3 items=["no dialog", "OK message", "continue or stop message", "OK message + warnings", "continue/stop + warnings"] ("type of dialog (OK msg:1)")
            n434 = property on="EOM Voltage (Ch. 3)" class="Slide (strict)"() -> ("Value"=w1037:dbl)  [unwired: 2 in, 2 out]
            n435 = property on="X" class="Slide (strict)"() -> ("Value"=w1046:dbl)  [unwired: 2 in, 2 out]
            n436 = property on="Y" class="Slide (strict)"() -> ("Value"=w1047:dbl)  [unwired: 2 in, 2 out]
            n437 = call-poly <vilib>:"DAQmx Create Virtual Channel.vi"("lines"=w1036, "line grouping"=w1030) -> ("task out"=w1035:refnum<k21>, "error out"=w1034:errorcluster)  [unwired: 12 in]
            n438 = call-poly <vilib>:"DAQmx Create Virtual Channel.vi"("maximum value"=w1044, "minimum value"=w1043, "physical channels"=w1042) -> ("task out"=w1051:refnum<k21>, "error out"=w1052:errorcluster)  [unwired: 11 in]
            n439 = Build Array(w1046, w1047, w1037, 0.0 ("element")) -> (w1045:dbl[])
            n440 = call-poly <vilib>:"DAQmx Write.vi"("task/channels in"=w1051, "data"=w1045, "timeout"=10.0, "error in"=w1052) -> ("task out"=w1048:refnum<k21>, "error out"=w1049:errorcluster)  [unwired: 9 in, 1 out]
            n441 = call-poly <vilib>:"DAQmx Write.vi"("task/channels in"=w1035, "data"=bool[] [FALSE, FALSE], "error in"=w1034) -> ("task out"=w1032:refnum<k21>, "error out"=w1033:errorcluster)  [unwired: 10 in, 1 out]
            n442 = call <vilib>:"DAQmx Clear Task.vi"("task in"=w1048, "error in"=w1049) -> ("error out"=w1040:errorcluster)  [unwired: 13 in]
            n443 = call <vilib>:"DAQmx Clear Task.vi"("task in"=w1032, "error in"=w1033) -> ("error out"=w1031:errorcluster)  [unwired: 13 in]
            n444 = call <vilib>:"Simple Error Handler.vi"("error in (no error)"=w1031) -> ()  [unwired: 4 in, 5 out]
            n445 = call <vilib>:"Simple Error Handler.vi"("type of dialog (OK msg:1)"=w1039, "error in (no error)"=w1040) -> ()  [unwired: 3 in, 5 out]
            "Direction" <- w1038
          }
        }
        n446 = property on="Focus Position?" class="Bool (strict)"("Value"=w994) -> ()  [unwired: 2 in, 2 out]
        n447 = property on="Lock Z" class="Bool (strict)"("Value"=w994) -> ()  [unwired: 2 in, 2 out]
        n448 = property on="Notification" class="Ring (strict)"("Value"=w991) -> ()  [unwired: 2 in, 2 out]
      }
      event "stop": Value Change {
        w1058 = u16 0 items=["", "North", "East", "South", "West"] ("Direction")
        w1053 = FALSE ("Focus Position?")
        n449 = event-data() -> ()  [unwired: 1 in, 5 out]
        n450 = flat-sequence {
          tunnel: w1062 -> [w1071]
          tunnel: w1057 -> [w1067]
          tunnel: w1056 -> [w1066]
          tunnel: w1055 -> [w1065]
          tunnel: w1061 -> [w1106]
          tunnel: w1060 -> [w1105]
          tunnel: w1059 -> [w1104]
          tunnel: w1054 -> [w1093]
          frame #0 {
            n451 = property on="Synced Trigger?" class="Bool (strict)"() -> ("Value"=w1064:bool)  [unwired: 2 in, 2 out]
            n452 = property on="Spinning" class="Bool (strict)"() -> ("Value"=w1069:bool)  [unwired: 2 in, 2 out]
            n453 = property on="Quivering" class="Bool (strict)"() -> ("Value"=w1070:bool)  [unwired: 2 in, 2 out]
            n454 = Or(x=w1069, y=w1070) -> (x .or. y?=w1068:bool)
            n455 = case shown="True" w1068 {
              tunnel: w1071 -> [_ w1078]
              tunnel: w1067 -> [_ w1076]
              tunnel: w1066 -> [_ w1075]
              tunnel: w1065 -> [_ w1074]
              tunnel: w1064 -> [_ w1072]
              frame False {
              }
              frame True {
                w1077 = FALSE ("Spinning")
                w1082 = T3 3 items=["no dialog", "OK message", "continue or stop message", "OK message + warnings", "continue/stop + warnings"] ("type of dialog (OK msg:1)")
                n456 = case shown="False" w1072 {
                  tunnel: w1076 -> [_ w1092]
                  tunnel: w1075 -> [_ w1091]
                  tunnel: w1074 -> [w1083 w1090]
                  tunnel: [w1083 w1084] -> w1073
                  frame False {
                  }
                  frame True {
                    n457 = call <vilib>:"DAQmx Is Task Done.vi"("task/channels in"=w1092, "error in"=w1090) -> ("task out"=w1085:refnum<k21>, "error out"=w1089:errorcluster)  [unwired: 11 in, 1 out]
                    n458 = call <vilib>:"DAQmx Is Task Done.vi"("task/channels in"=w1091, "error in"=w1089) -> ("task out"=w1087:refnum<k21>, "error out"=w1088:errorcluster)  [unwired: 11 in, 1 out]
                    n459 = call <vilib>:"DAQmx Clear Task.vi"("task in"=w1087, "error in"=w1088) -> ("error out"=w1086:errorcluster)  [unwired: 13 in]
                    n460 = call <vilib>:"DAQmx Clear Task.vi"("task in"=w1085, "error in"=w1086) -> ("error out"=w1084:errorcluster)  [unwired: 13 in]
                  }
                }
                n461 = property on="Spinning" class="Bool (strict)"("Value"=w1077) -> ()  [unwired: 2 in, 2 out]
                n462 = property on="Quivering" class="Bool (strict)"("Value"=w1077) -> ()  [unwired: 2 in, 2 out]
                n463 = call <vilib>:"DAQmx Is Task Done.vi"("task/channels in"=w1078, "error in"=w1073) -> ("task out"=w1079:refnum<k21>, "error out"=w1080:errorcluster)  [unwired: 11 in, 1 out]
                n464 = call <vilib>:"DAQmx Clear Task.vi"("task in"=w1079, "error in"=w1080) -> ("error out"=w1081:errorcluster)  [unwired: 13 in]
                n465 = call <vilib>:"Simple Error Handler.vi"("type of dialog (OK msg:1)"=w1082, "error in (no error)"=w1081) -> ()  [unwired: 3 in, 5 out]
              }
            }
          }
          frame #1 {
            w1095 = 0 items=["one channel for each line", "one channel for all lines"] ("line grouping")
            w1101 = T3 3 items=["no dialog", "OK message", "continue or stop message", "OK message + warnings", "continue/stop + warnings"] ("type of dialog (OK msg:1)")
            w1103 = 0.0 ("element")
            n466 = call-poly <vilib>:"DAQmx Create Virtual Channel.vi"("lines"=w1093, "line grouping"=w1095) -> ("task out"=w1100:refnum<k21>, "error out"=w1099:errorcluster)  [unwired: 12 in]
            n467 = call-poly <vilib>:"DAQmx Create Virtual Channel.vi"("maximum value"=w1105, "minimum value"=w1104, "physical channels"=w1106) -> ("task out"=w1111:refnum<k21>, "error out"=w1112:errorcluster)  [unwired: 11 in]
            n468 = Build Array(w1103, w1103, w1103, w1103) -> (w1107:dbl[])
            n469 = call-poly <vilib>:"DAQmx Write.vi"("task/channels in"=w1111, "data"=w1107, "timeout"=10.0, "error in"=w1112) -> ("task out"=w1108:refnum<k21>, "error out"=w1109:errorcluster)  [unwired: 9 in, 1 out]
            n470 = call-poly <vilib>:"DAQmx Write.vi"("task/channels in"=w1100, "data"=bool[] [FALSE, FALSE], "error in"=w1099) -> ("task out"=w1097:refnum<k21>, "error out"=w1098:errorcluster)  [unwired: 10 in, 1 out]
            n471 = call <vilib>:"DAQmx Clear Task.vi"("task in"=w1108, "error in"=w1109) -> ("error out"=w1102:errorcluster)  [unwired: 13 in]
            n472 = call <vilib>:"DAQmx Clear Task.vi"("task in"=w1097, "error in"=w1098) -> ("error out"=w1096:errorcluster)  [unwired: 13 in]
            n473 = call <vilib>:"Simple Error Handler.vi"("error in (no error)"=w1096) -> ()  [unwired: 4 in, 5 out]
            n474 = call <vilib>:"Simple Error Handler.vi"("type of dialog (OK msg:1)"=w1101, "error in (no error)"=w1102) -> ()  [unwired: 3 in, 5 out]
          }
        }
        n475 = property on="Lock Z" class="Bool (strict)"("Value"=w1053) -> ()  [unwired: 2 in, 2 out]
        n476 = property on="Focus Position?" class="Bool (strict)"("Value"=w1053) -> ()  [unwired: 2 in, 2 out]
        n477 = property on="Laser Trig 1" class="Bool (strict)"("Value"=w1053) -> ()  [unwired: 2 in, 2 out]
        n478 = property on="Direction" class="Ring (strict)"("Value"=w1058) -> ()  [unwired: 2 in, 2 out]
      }
    }
    n479 = property on="Center" class="Bool (strict)"("Value"=w19) -> ()  [unwired: 2 in, 2 out]
    n480 = property on="Stop spin" class="Bool (strict)"("Value"=w21) -> ()  [unwired: 2 in, 2 out]
    n481 = property on="Spin" class="Bool (strict)"("Value"=w20) -> ()  [unwired: 2 in, 2 out]
    n482 = property on="Scan Galvo" class="Bool (strict)"("Value"=w38) -> ()  [unwired: 2 in, 2 out]
    n483 = property on="2D Center Find" class="Bool (strict)"("Value"=w32) -> ()  [unwired: 2 in, 2 out]
    n484 = property on="Quiver" class="Bool (strict)"("Value"=w11) -> ()  [unwired: 2 in, 2 out]
    n485 = property on="North" class="Bool (strict)"("Value"=w15) -> ()  [unwired: 2 in, 2 out]
    n486 = property on="West" class="Bool (strict)"("Value"=w16) -> ()  [unwired: 2 in, 2 out]
    n487 = property on="South" class="Bool (strict)"("Value"=w17) -> ()  [unwired: 2 in, 2 out]
    n488 = property on="East" class="Bool (strict)"("Value"=w18) -> ()  [unwired: 2 in, 2 out]
  }
  n489 = while {
    stop <- w1115 stop-if-true
    n490 = event shown="[1] \"Focus Position?\": Value Change" {
      selector: _ -> [_ _ _]
      dyn-events: _ -> [_ _ _]
      timeout: _ -> [_ _ _]
      tunnel: [_ _ w1256] -> w1115
      tunnel: [w1116 _ _] -> w1114
      tunnel: [_ w1216 _] -> w1113
      event "Lock Z": Value Change {
        n491 = event-data() -> ()  [unwired: 1 in, 5 out]
        n492 = property on="Spinning" class="Bool (strict)"() -> ("Value"=w1117:bool)  [unwired: 2 in, 2 out]
        n493 = case shown="True" w1117 {
          tunnel: [FALSE ("Value") w1123] -> w1116
          frame False {
            w1120 = u16 1 items=["", "Spin must be activated for focus lock"] ("Text Ring 2")
            n494 = property on="Lock Z" class="Bool (strict)"("Value"=FALSE) -> ()  [unwired: 2 in, 2 out]
            "Notification" <- w1120
          }
          frame True {
            w1136 = u16 0 items=["", "Active spin for focus lock"] ("Text Ring 2")
            w1155 = 2 ("Device Number (1)")
            n495 = call <instrlib>:"Initialize.vi"("VISA Resource Name"="IX2-UCB port") -> ("VISA Resource Name Out"=w1160:refnum<visa-resource-name>, "error out"=w1161:errorcluster)  [unwired: 13 in]
            n496 = Divide(x="Focus limit width", y=2.0) -> (x/y=w1127:dbl)
            n497 = call-poly <vilib>:"DAQmx Create Virtual Channel.vi"("physical channels"="Lock-in Amp In") -> ("task out"=w1148:refnum<k21>, "error out"=w1149:errorcluster)  [unwired: 13 in]
            n498 = Add(x=w1127, y="Focus Limit Center") -> (x+y=w1126:dbl)
            n499 = Subtract(x="Focus Limit Center", y=w1127) -> (x-y=w1125:dbl)
            n500 = call <instrlib>:"Login Device.vi"("error in (no error)"=w1161, "Device Number (1)"=w1155, "VISA Resource Name"=w1160) -> ("error out"=w1158:errorcluster, "VISA Resource Name Out"=w1157:refnum<visa-resource-name>)  [unwired: 7 in]
            n501 = property on="Notification" class="Ring (strict)"("Value"=w1136) -> ()  [unwired: 2 in, 2 out]
            n502 = call <vilib>:"DAQmx Start Task.vi"("task/channels in"=w1148, "error in"=w1149) -> ("task out"=w1146:refnum<k21>, "error out"=w1147:errorcluster)  [unwired: 12 in]
            n503 = call <instrlib>:"Set Software Limits.vi"("VISA Resource Name"=w1157, "Device Number (1)"=w1155, "Near Limit (30000.0 um)"=w1126, "Far Limit (0.01 um)"=w1125, "error in (no error)"=w1158) -> ("VISA Resource Name Out"=w1156:refnum<visa-resource-name>, "error out"=w1154:errorcluster)  [unwired: 9 in]
            n504 = flat-sequence {
              tunnel: w1146 -> [w1169]
              tunnel: w1147 -> [w1168]
              tunnel: w1154 -> [w1165]
              tunnel: w1155 -> [w1163]
              tunnel: w1156 -> [w1162]
              tunnel: [w1162] -> w1135
              tunnel: [w1165] -> w1134
              tunnel: [w1166] -> w1133
              tunnel: [w1167] -> w1132
              tunnel: [w1163] -> w1131
              tunnel: [w1184] -> w1145
              tunnel: [w1183] -> w1143
              tunnel: [w1182] -> w1142
              tunnel: [w1181] -> w1141
              tunnel: [w1180] -> w1139
              tunnel: w1135 -> [w1188]
              tunnel: w1134 -> [w1187]
              tunnel: w1133 -> [w1186]
              tunnel: w1132 -> [w1185]
              tunnel: w1131 -> [w1179]
              tunnel: [w1178] -> w1123
              tunnel: [w1177] -> w1121
              frame #0 {
                n505 = case shown="True" "Use current position?" {
                  tunnel: w1169 -> [w1171 w1176]
                  tunnel: w1168 -> [w1170 w1173]
                  tunnel: [w1171 w1175] -> w1167
                  tunnel: [w1170 w1174] -> w1166
                  frame False {
                  }
                  frame True {
                    n506 = call-poly <vilib>:"DAQmx Read.vi"("task/channels in"=w1176, "error in"=w1173) -> ("task out"=w1175:refnum<k21>, "data"=w1172:dbl, "error out"=w1174:errorcluster)  [unwired: 11 in]
                    n507 = property on="Z lock setpoint (Volt)" class="Slide (strict)"("Value"=w1172) -> ()  [unwired: 2 in, 2 out]
                  }
                }
              }
              frame #1 {
                n508 = while {
                  tunnel: w1188 -> [w1198]
                  tunnel: w1179 -> [w1201]
                  tunnel: w1187 -> [w1197]
                  tunnel: [w1208] -> w1181
                  tunnel: [w1212] -> w1180
                  tunnel: w1186 -> [w1205]
                  tunnel: w1185 -> [w1204]
                  tunnel: [w1203] -> w1184
                  tunnel: [w1202] -> w1183
                  tunnel: [w1201] -> w1182
                  tunnel: [w1193] -> w1178
                  tunnel: [w1189] -> w1177 mode=indexing
                  stop <- w1209 stop-if-true
                  n509 = call-poly <vilib>:"DAQmx Read.vi"("task/channels in"=w1204, "error in"=w1205) -> ("task out"=w1202:refnum<k21>, "data"=w1189:dbl, "error out"=w1203:errorcluster)  [unwired: 11 in]
                  n510 = Wait (ms)(milliseconds to wait="Sampling Time") -> ()  [unwired: 1 out]
                  n511 = call-poly <vilib>:"PID Advanced.vi"("setpoint"="Z lock setpoint (Volt)", "output range"="output range", "process variable"=w1189, "setpoint range"="setpoint range", "PID gains"="PID gains", "dt (s)"="Sampling Time") -> ("output"=w1199:dbl)  [unwired: 8 in, 1 out]
                  n512 = Absolute Value(x=w1199) -> (abs(x)=w1200:dbl)
                  n513 = Less Than 0?(x=w1199) -> (x < 0?=w1211:bool)
                  n514 = property on="Focus Position?" class="Bool (strict)"() -> ("Value"=w1193:bool)  [unwired: 2 in, 2 out]
                  n515 = case shown="True" w1211 {
                    tunnel: [enum16{"Up", "Down"}."Up" ("Direction (1: Down)") enum16{"Up", "Down"}."Down" ("Direction (1: Down)")] -> w1210
                    frame False {
                    }
                    frame True {
                    }
                  }
                  n516 = Unbundle By Name(w1203) -> ("status"=w1207:bool)
                  n517 = Not(x="Lock Z") -> (.not. x?=w1195:bool)
                  n518 = call <instrlib>:"Move Focusing Unit.vi"("VISA Resource Name"=w1198, "Device Number (1)"=w1201, "Direction (1: Down)"=w1210, "Step (0.0 um)"=w1200, "error in (no error)"=w1197) -> ("VISA Resource Name Out"=w1212:refnum<visa-resource-name>, "error out"=w1208:errorcluster)  [unwired: 9 in]
                  n519 = Unbundle By Name(w1208) -> ("status"=w1206:bool)
                  n520 = Compound Arithmetic op=OR(w1206, w1207, w1195, w1193) -> (w1209:bool)
                }
              }
            }
            n521 = call <instrlib>:"Error Message.vi"("VISA Resource Name"=w1139, "error in (no error)"=w1141) -> ("VISA Resource Name Out"=w1138:refnum<visa-resource-name>, "error out"=w1140:errorcluster)  [unwired: 9 in, 3 out]
            n522 = call <instrlib>:"Logout Device.vi"("error in (no error)"=w1140, "Device Number (1)"=w1142, "VISA Resource Name"=w1138) -> ("error out"=w1153:errorcluster, "VISA Resource Name Out"=w1152:refnum<visa-resource-name>)  [unwired: 7 in]
            n523 = property on="Focus Position?" class="Bool (strict)"("Value"=FALSE ("Focus Position?")) -> ()  [unwired: 2 in, 2 out]
            n524 = call <vilib>:"DAQmx Clear Task.vi"("task in"=w1143, "error in"=w1145) -> ("error out"=w1144:errorcluster)  [unwired: 13 in]
            n525 = call <instrlib>:"Error Message.vi"("VISA Resource Name"=w1152, "error in (no error)"=w1153) -> ("VISA Resource Name Out"=w1150:refnum<visa-resource-name>, "error out"=w1151:errorcluster)  [unwired: 9 in, 3 out]
            n526 = call <instrlib>:"Close.vi"("VISA Resource Name"=w1150, "error in (no error)"=w1151) -> ("error out"=w1137:errorcluster)  [unwired: 13 in]
            n527 = call <vilib>:"Simple Error Handler.vi"("error in (no error)"=w1144) -> ()  [unwired: 4 in, 5 out]
            n528 = call <vilib>:"Simple Error Handler.vi"("error in (no error)"=w1137) -> ()  [unwired: 4 in, 5 out]
            "Array" <- w1121
          }
        }
      }
      event "Focus Position?": Value Change {
        n529 = event-data() -> ()  [unwired: 1 in, 5 out]
        n530 = property on="Spinning" class="Bool (strict)"() -> ("Value"=w1218:bool)  [unwired: 2 in, 2 out]
        n531 = case shown="True" w1218 {
          tunnel: [FALSE ("Value") w1222] -> w1216
          frame False {
            w1221 = u16 2 items=["", "Spin must be activated for focus lock", "Spin must be activated for focus detection"] ("Notification")
            n532 = property on="Notification" class="Ring (strict)"("Value"=w1221) -> ()  [unwired: 2 in, 2 out]
            n533 = property on="Focus Position?" class="Bool (strict)"("Value"=FALSE ("Focus Position?")) -> ()  [unwired: 2 in, 2 out]
          }
          frame True {
            n534 = while {
              tunnel: [w1225] -> w1222
              stop <- w1229 stop-if-true
              w1238 = 2 ("Device Number (1)")
              n535 = property on="Lock-in Amp In" class="DAQmxName"() -> ("Value"=w1223:string)  [unwired: 2 in, 2 out]
              n536 = call-poly <vilib>:"DAQmx Create Virtual Channel.vi"("physical channels"=w1223) -> ("task out"=w1254:refnum<k21>, "error out"=w1255:errorcluster)  [unwired: 13 in]
              n537 = property on="IX2-UCB port" class="VISAName"() -> ("Value"=w1237:refnum<visa-resource-name>)  [unwired: 2 in, 2 out]
              n538 = call <vilib>:"DAQmx Start Task.vi"("task/channels in"=w1254, "error in"=w1255) -> ("task out"=w1253:refnum<k21>, "error out"=w1252:errorcluster)  [unwired: 12 in]
              n539 = call <instrlib>:"Initialize.vi"("VISA Resource Name"=w1237) -> ("VISA Resource Name Out"=w1249:refnum<visa-resource-name>)  [unwired: 13 in, 1 out]
              n540 = call-poly <vilib>:"DAQmx Read.vi"("task/channels in"=w1253, "error in"=w1252) -> ("task out"=w1250:refnum<k21>, "data"=w1227:dbl, "error out"=w1235:errorcluster)  [unwired: 11 in]
              n541 = Wait (ms)(milliseconds to wait=u32 100) -> ()  [unwired: 1 out]
              n542 = call <instrlib>:"Login Device.vi"("Device Number (1)"=w1238, "VISA Resource Name"=w1249) -> ("error out"=w1247:errorcluster, "VISA Resource Name Out"=w1248:refnum<visa-resource-name>)  [unwired: 8 in]
              n543 = call <instrlib>:"Get Focus Position.vi"("VISA Resource Name"=w1248, "Device Number (1)"=w1238, "error in (no error)"=w1247) -> ("VISA Resource Name Out"=w1239:refnum<visa-resource-name>, "position (um)"=w1228:dbl, "error out"=w1234:errorcluster)  [unwired: 10 in]
              n544 = Bundle("data"=w1227, "position (um)"=w1228, "element"=0.0) -> (→"position (um)":T1)  [unwired: 1 in]
              n545 = Unbundle By Name(w1235) -> ("status"=w1233:bool)
              n546 = Unbundle By Name(w1234) -> ("status"=w1232:bool)
              n547 = property on="Lock Z" class="Bool (strict)"() -> ("Value"=w1225:bool)  [unwired: 2 in, 2 out]
              n548 = call <instrlib>:"Error Message.vi"("VISA Resource Name"=w1239, "error in (no error)"=w1234) -> ("VISA Resource Name Out"=w1241:refnum<visa-resource-name>, "error out"=w1242:errorcluster)  [unwired: 9 in, 3 out]
              n549 = call <vilib>:"DAQmx Clear Task.vi"("task in"=w1250, "error in"=w1235) -> ("error out"=w1251:errorcluster)  [unwired: 13 in]
              n550 = Not(x="Focus Position?") -> (.not. x?=w1231:bool)
              n551 = call <instrlib>:"Logout Device.vi"("error in (no error)"=w1242, "Device Number (1)"=w1238, "VISA Resource Name"=w1241) -> ("error out"=w1246:errorcluster, "VISA Resource Name Out"=w1245:refnum<visa-resource-name>)  [unwired: 7 in]
              n552 = call <vilib>:"Simple Error Handler.vi"("error in (no error)"=w1251) -> ()  [unwired: 4 in, 5 out]
              n553 = call <instrlib>:"Error Message.vi"("VISA Resource Name"=w1245, "error in (no error)"=w1246) -> ("VISA Resource Name Out"=w1243:refnum<visa-resource-name>, "error out"=w1244:errorcluster)  [unwired: 9 in, 3 out]
              n554 = Compound Arithmetic op=OR(w1233, w1232, w1231, w1225) -> (w1229:bool)
              n555 = call <instrlib>:"Close.vi"("VISA Resource Name"=w1243, "error in (no error)"=w1244) -> ("error out"=w1240:errorcluster)  [unwired: 13 in]
              n556 = call <vilib>:"Simple Error Handler.vi"("error in (no error)"=w1240) -> ()  [unwired: 4 in, 5 out]
            }
          }
        }
        n557 = property on="Lock Z" class="Bool (strict)"("Value"=FALSE ("Lock Z")) -> ()  [unwired: 2 in, 2 out]
      }
      event "stop": Value Change {
        n558 = event-data() -> ()  [unwired: 1 in, 5 out]
        n559 = property on="stop" class="Bool (strict)"() -> ("Value"=w1256:bool)  [unwired: 2 in, 2 out]
      }
    }
    n560 = property on="Focus Position?" class="Bool (strict)"("Value"=w1114) -> ()  [unwired: 2 in, 2 out]
    n561 = property on="Lock Z" class="Bool (strict)"("Value"=w1113) -> ()  [unwired: 2 in, 2 out]
  }
